vi "TCam_Calibration.vi"() -> (2 "State out":string="Data: Load Thermal Calibration")   [LabVIEW 2020]
uses:
  DataCluster_TCAL.ctl
  <vilib>/vision/Image Controls.llb/IMAQ Image.ctl
  DataCluster.ctl
  <vilib>/userDefined/High Color/IMAQdx.ctl
  <vilib>/Utility/xml.llb/Write to XML File(string).vi
panel:
  out "Pict Ring":i32(ring)
  in  "Done":bool
  out "Step":string="Step: 4\n\nCalculate temperature!"
  in  "Fixpoint Radius":i32=20 min=3 max=20
  in  "Cluster":T1 {"Points"."Top Left"."Y" format="%.2f"; "Points"."Top Left"."X" format="%.2f"; "Points"."Top Right"."Y" format="%.2f"; "Points"."Top Right"."X" format="%.2f"; "Points"."Bottom Left"."Y" format="%.2f"; "Points"."Bottom Left"."X" format="%.2f"; "Points"."Bottom Right"."Y" format="%.2f"; "Points"."Bottom Right"."X" format="%.2f"; "Points"."Fixpoint"."Y" format="%.2f"; "Points"."Fixpoint"."X" format="%.2f"}
  in  "Display Mapping":u32(ring)=10 items=["Default"=10, "Most Significant Bits"=11, "Full Dynamic"=12, "Downshift"=13, "Given Range"=14, "90% Dynamic"=15, "Given Percent Range"=16]
  in  "Image":u32(slide) scale=0.0..242.0
  in  "Help":bool
  out "Tutorial":string="Step: 4\n\nCalculate temperature!"
  in  "Show All Points":bool
  in  "Well Radius":u32=50 min=1 max=100
  in  "PCR Size":u16(ring) items=["384 (24x16)", "96 (12x8)"]
  out "Points":T3[](array[typedef])=[{"X"=103.0, "Y"=94.0}, {"X"=158.04349, "Y"=93.521736}, {"X"=213.08696, "Y"=93.04348}, {"X"=268.13043, "Y"=92.565216}, {"X"=323.17392, "Y"=92.08696}, {"X"=378.2174, "Y"=91.608696}, {"X"=433.26086, "Y"=91.13043}, {"X"=488.30435, "Y"=90.652176}, {"X"=543.34784, "Y"=90.17391}, {"X"=598.39136, "Y"=89.69565}, {"X"=653.4348, "Y"=89.21739}, {"X"=708.4783, "Y"=88.73913}, {"X"=763.5217, "Y"=88.26087}, {"X"=818.56525, "Y"=87.78261}, {"X"=873.6087, "Y"=87.30435}, {"X"=928.6522, "Y"=86.82609}, {"X"=983.6957, "Y"=86.347824}, {"X"=1038.7391, "Y"=85.86957}, {"X"=1093.7827, "Y"=85.391304}, {"X"=1148.8262, "Y"=84.91304}, {"X"=1203.8696, "Y"=84.434784}, {"X"=1258.9131, "Y"=83.95652}, {"X"=1313.9565, "Y"=83.478264}, {"X"=1369.0, "Y"=83.0}, {"X"=103.46667, "Y"=149.06667}, {"X"=158.51015, "Y"=148.58841}, {"X"=213.55362, "Y"=148.11014}, {"X"=268.5971, "Y"=147.63188}, {"X"=323.6406, "Y"=147.15363}, {"X"=378.68408, "Y"=146.67535}, {"X"=433.72754, "Y"=146.1971}, {"X"=488.77103, "Y"=145.71884}, {"X"=543.8145, "Y"=145.24057}, {"X"=598.858, "Y"=144.76231}, {"X"=653.9015, "Y"=144.28406}, {"X"=708.94495, "Y"=143.8058}, {"X"=763.9884, "Y"=143.32753}, {"X"=819.0319, "Y"=142.84927}, {"X"=874.0754, "Y"=142.37102}, {"X"=929.1189, "Y"=141.89276}, {"X"=984.16235, "Y"=141.41449}, {"X"=1039.2058, "Y"=140.93623}, {"X"=1094.2493, "Y"=140.45798}, {"X"=1149.2928, "Y"=139.9797}, {"X"=1204.3363, "Y"=139.50145}, {"X"=1259.3798, "Y"=139.0232}, {"X"=1314.4232, "Y"=138.54492}, {"X"=1369.4667, "Y"=138.06667}, {"X"=103.933334, "Y"=204.13333}, {"X"=158.9768, "Y"=203.65506}, {"X"=214.0203, "Y"=203.17682}, {"X"=269.06375, "Y"=202.69855}, {"X"=324.10724, "Y"=202.22029}, {"X"=379.15073, "Y"=201.74203}, {"X"=434.19418, "Y"=201.26376}, {"X"=489.23767, "Y"=200.7855}, {"X"=544.2812, "Y"=200.30725}, {"X"=599.32465, "Y"=199.82898}, {"X"=654.36816, "Y"=199.35072}, {"X"=709.4116, "Y"=198.87247}, {"X"=764.4551, "Y"=198.3942}, {"X"=819.4986, "Y"=197.91594}, {"X"=874.54205, "Y"=197.43768}, {"X"=929.5856, "Y"=196.95941}, {"X"=984.629, "Y"=196.48116}, {"X"=1039.6725, "Y"=196.0029}, {"X"=1094.716, "Y"=195.52463}, {"X"=1149.7595, "Y"=195.04637}, {"X"=1204.803, "Y"=194.56812}, {"X"=1259.8464, "Y"=194.08984}, {"X"=1314.8899, "Y"=193.6116}, {"X"=1369.9333, "Y"=193.13333}, {"X"=104.4, "Y"=259.2}, {"X"=159.44348, "Y"=258.72174}, {"X"=214.48695, "Y"=258.24347}, {"X"=269.53043, "Y"=257.7652}, {"X"=324.5739, "Y"=257.28696}, {"X"=379.6174, "Y"=256.8087}, {"X"=434.66086, "Y"=256.33044}, {"X"=489.70435, "Y"=255.85217}, {"X"=544.74786, "Y"=255.37392}, {"X"=599.7913, "Y"=254.89565}, {"X"=654.83484, "Y"=254.41739}, {"X"=709.8783, "Y"=253.93913}, {"X"=764.92175, "Y"=253.46086}, {"X"=819.9653, "Y"=252.9826}, {"X"=875.0087, "Y"=252.50435}, {"X"=930.05225, "Y"=252.02608}, {"X"=985.0957, "Y"=251.54782}, {"X"=1040.1392, "Y"=251.06956}, {"X"=1095.1826, "Y"=250.59131}, {"X"=1150.2262, "Y"=250.11304}, {"X"=1205.2697, "Y"=249.63478}, {"X"=1260.3131, "Y"=249.15652}, {"X"=1315.3566, "Y"=248.67825}, {"X"=1370.4, "Y"=248.2}, {"X"=104.86667, "Y"=314.26666}, {"X"=159.91014, "Y"=313.7884}, {"X"=214.95363, "Y"=313.31012}, {"X"=269.9971, "Y"=312.83188}, {"X"=325.0406, "Y"=312.35364}, {"X"=380.08408, "Y"=311.87537}, {"X"=435.12753, "Y"=311.3971}, {"X"=490.17102, "Y"=310.91882}, {"X"=545.2145, "Y"=310.44058}, {"X"=600.258, "Y"=309.9623}, {"X"=655.30145, "Y"=309.48407}, {"X"=710.3449, "Y"=309.0058}, {"X"=765.38837, "Y"=308.52753}, {"X"=820.4319, "Y"=308.04926}, {"X"=875.47534, "Y"=307.571}, {"X"=930.51886, "Y"=307.09274}, {"X"=985.5623, "Y"=306.6145}, {"X"=1040.6058, "Y"=306.13623}, {"X"=1095.6493, "Y"=305.65796}, {"X"=1150.6929, "Y"=305.1797}, {"X"=1205.7363, "Y"=304.70145}, {"X"=1260.7798, "Y"=304.2232}, {"X"=1315.8232, "Y"=303.74493}, {"X"=1370.8667, "Y"=303.26666}, {"X"=105.333336, "Y"=369.3333}, {"X"=160.37682, "Y"=368.85504}, {"X"=215.42029, "Y"=368.3768}, {"X"=270.46378, "Y"=367.89853}, {"X"=325.50726, "Y"=367.42026}, {"X"=380.55075, "Y"=366.94202}, {"X"=435.5942, "Y"=366.46375}, {"X"=490.6377, "Y"=365.98547}, {"X"=545.68115, "Y"=365.50723}, {"X"=600.7247, "Y"=365.02896}, {"X"=655.7681, "Y"=364.5507}, {"X"=710.8116, "Y"=364.07245}, {"X"=765.85504, "Y"=363.59418}, {"X"=820.89856, "Y"=363.11594}, {"X"=875.942, "Y"=362.63766}, {"X"=930.98553, "Y"=362.1594}, {"X"=986.029, "Y"=361.68115}, {"X"=1041.0725, "Y"=361.20288}, {"X"=1096.116, "Y"=360.7246}, {"X"=1151.1595, "Y"=360.24637}, {"X"=1206.203, "Y"=359.7681}, {"X"=1261.2465, "Y"=359.28983}, {"X"=1316.2899, "Y"=358.81158}, {"X"=1371.3334, "Y"=358.3333}, {"X"=105.8, "Y"=424.4}, {"X"=160.84348, "Y"=423.92172}, {"X"=215.88696, "Y"=423.44348}, {"X"=270.93042, "Y"=422.9652}, {"X"=325.9739, "Y"=422.48694}, {"X"=381.0174, "Y"=422.0087}, {"X"=436.06085, "Y"=421.53043}, {"X"=491.10434, "Y"=421.05215}, {"X"=546.1478, "Y"=420.5739}, {"X"=601.19135, "Y"=420.09564}, {"X"=656.2348, "Y"=419.61737}, {"X"=711.27826, "Y"=419.13913}, {"X"=766.3217, "Y"=418.66086}, {"X"=821.36523, "Y"=418.18262}, {"X"=876.4087, "Y"=417.70435}, {"X"=931.4522, "Y"=417.22607}, {"X"=986.49567, "Y"=416.74783}, {"X"=1041.5392, "Y"=416.26956}, {"X"=1096.5826, "Y"=415.7913}, {"X"=1151.6262, "Y"=415.31305}, {"X"=1206.6697, "Y"=414.83478}, {"X"=1261.7131, "Y"=414.3565}, {"X"=1316.7566, "Y"=413.87827}, {"X"=1371.8, "Y"=413.4}, {"X"=106.26667, "Y"=479.46667}, {"X"=161.31015, "Y"=478.9884}, {"X"=216.35362, "Y"=478.51016}, {"X"=271.3971, "Y"=478.0319}, {"X"=326.44058, "Y"=477.55362}, {"X"=381.48407, "Y"=477.07538}, {"X"=436.52753, "Y"=476.5971}, {"X"=491.571, "Y"=476.11884}, {"X"=546.6145, "Y"=475.6406}, {"X"=601.658, "Y"=475.16232}, {"X"=656.7015, "Y"=474.68405}, {"X"=711.74493, "Y"=474.2058}, {"X"=766.7884, "Y"=473.72754}, {"X"=821.8319, "Y"=473.2493}, {"X"=876.87537, "Y"=472.77103}, {"X"=931.9189, "Y"=472.29276}, {"X"=986.96234, "Y"=471.8145}, {"X"=1042.0059, "Y"=471.33624}, {"X"=1097.0493, "Y"=470.85797}, {"X"=1152.0929, "Y"=470.37973}, {"X"=1207.1364, "Y"=469.90146}, {"X"=1262.1798, "Y"=469.4232}, {"X"=1317.2233, "Y"=468.94495}, {"X"=1372.2667, "Y"=468.46667}, {"X"=106.73333, "Y"=534.5333}, {"X"=161.77681, "Y"=534.05505}, {"X"=216.8203, "Y"=533.5768}, {"X"=271.86377, "Y"=533.0985}, {"X"=326.90726, "Y"=532.62024}, {"X"=381.95074, "Y"=532.142}, {"X"=436.9942, "Y"=531.66376}, {"X"=492.0377, "Y"=531.1855}, {"X"=547.0812, "Y"=530.7073}, {"X"=602.12463, "Y"=530.229}, {"X"=657.16815, "Y"=529.75073}, {"X"=712.2116, "Y"=529.27246}, {"X"=767.25507, "Y"=528.7942}, {"X"=822.2986, "Y"=528.3159}, {"X"=877.34204, "Y"=527.83765}, {"X"=932.38556, "Y"=527.3594}, {"X"=987.429, "Y"=526.88116}, {"X"=1042.4724, "Y"=526.4029}, {"X"=1097.516, "Y"=525.9246}, {"X"=1152.5594, "Y"=525.4464}, {"X"=1207.6029, "Y"=524.96814}, {"X"=1262.6464, "Y"=524.48987}, {"X"=1317.6898, "Y"=524.0116}, {"X"=1372.7333, "Y"=523.5333}, {"X"=107.2, "Y"=589.6}, {"X"=162.24348, "Y"=589.1217}, {"X"=217.28696, "Y"=588.64343}, {"X"=272.33044, "Y"=588.16516}, {"X"=327.37393, "Y"=587.6869}, {"X"=382.41742, "Y"=587.2087}, {"X"=437.46088, "Y"=586.7304}, {"X"=492.50436, "Y"=586.25214}, {"X"=547.54785, "Y"=585.7739}, {"X"=602.5913, "Y"=585.29565}, {"X"=657.6348, "Y"=584.8174}, {"X"=712.6783, "Y"=584.3391}, {"X"=767.72174, "Y"=583.86084}, {"X"=822.76526, "Y"=583.38257}, {"X"=877.8087, "Y"=582.9043}, {"X"=932.85223, "Y"=582.426}, {"X"=987.8957, "Y"=581.9478}, {"X"=1042.9391, "Y"=581.46954}, {"X"=1097.9827, "Y"=580.9913}, {"X"=1153.0261, "Y"=580.51306}, {"X"=1208.0696, "Y"=580.0348}, {"X"=1263.113, "Y"=579.5565}, {"X"=1318.1565, "Y"=579.07825}, {"X"=1373.2, "Y"=578.6}, {"X"=107.666664, "Y"=644.6666}, {"X"=162.71014, "Y"=644.18835}, {"X"=217.75363, "Y"=643.7101}, {"X"=272.7971, "Y"=643.2319}, {"X"=327.84058, "Y"=642.7536}, {"X"=382.88406, "Y"=642.2753}, {"X"=437.92752, "Y"=641.79706}, {"X"=492.971, "Y"=641.3188}, {"X"=548.0145, "Y"=640.8405}, {"X"=603.058, "Y"=640.3623}, {"X"=658.1015, "Y"=639.88403}, {"X"=713.14496, "Y"=639.40576}, {"X"=768.1884, "Y"=638.9275}, {"X"=823.23193, "Y"=638.4492}, {"X"=878.2754, "Y"=637.97095}, {"X"=933.3189, "Y"=637.49274}, {"X"=988.36237, "Y"=637.01447}, {"X"=1043.4058, "Y"=636.5362}, {"X"=1098.4493, "Y"=636.0579}, {"X"=1153.4928, "Y"=635.57965}, {"X"=1208.5363, "Y"=635.1014}, {"X"=1263.5797, "Y"=634.62317}, {"X"=1318.6232, "Y"=634.1449}, {"X"=1373.6666, "Y"=633.6666}, {"X"=108.13333, "Y"=699.73334}, {"X"=163.17682, "Y"=699.25507}, {"X"=218.22029, "Y"=698.7768}, {"X"=273.26376, "Y"=698.2986}, {"X"=328.30725, "Y"=697.8203}, {"X"=383.35074, "Y"=697.34204}, {"X"=438.3942, "Y"=696.8638}, {"X"=493.43768, "Y"=696.3855}, {"X"=548.4812, "Y"=695.9072}, {"X"=603.52466, "Y"=695.429}, {"X"=658.5682, "Y"=694.95074}, {"X"=713.61163, "Y"=694.4725}, {"X"=768.6551, "Y"=693.9942}, {"X"=823.6986, "Y"=693.5159}, {"X"=878.74207, "Y"=693.03766}, {"X"=933.7856, "Y"=692.55945}, {"X"=988.82904, "Y"=692.0812}, {"X"=1043.8724, "Y"=691.6029}, {"X"=1098.916, "Y"=691.12463}, {"X"=1153.9595, "Y"=690.64636}, {"X"=1209.0029, "Y"=690.1681}, {"X"=1264.0464, "Y"=689.6899}, {"X"=1319.0898, "Y"=689.2116}, {"X"=1374.1333, "Y"=688.73334}, {"X"=108.6, "Y"=754.8}, {"X"=163.64348, "Y"=754.3217}, {"X"=218.68697, "Y"=753.84344}, {"X"=273.73044, "Y"=753.36523}, {"X"=328.77393, "Y"=752.88696}, {"X"=383.8174, "Y"=752.4087}, {"X"=438.86087, "Y"=751.9304}, {"X"=493.90436, "Y"=751.45215}, {"X"=548.9478, "Y"=750.9739}, {"X"=603.99133, "Y"=750.49567}, {"X"=659.0348, "Y"=750.0174}, {"X"=714.07825, "Y"=749.5391}, {"X"=769.1217, "Y"=749.06085}, {"X"=824.1652, "Y"=748.5826}, {"X"=879.2087, "Y"=748.1043}, {"X"=934.2522, "Y"=747.6261}, {"X"=989.29565, "Y"=747.1478}, {"X"=1044.3391, "Y"=746.66956}, {"X"=1099.3827, "Y"=746.1913}, {"X"=1154.4261, "Y"=745.713}, {"X"=1209.4696, "Y"=745.23474}, {"X"=1264.5131, "Y"=744.75653}, {"X"=1319.5565, "Y"=744.27826}, {"X"=1374.6, "Y"=743.8}, {"X"=109.066666, "Y"=809.86664}, {"X"=164.11015, "Y"=809.38837}, {"X"=219.15363, "Y"=808.9101}, {"X"=274.1971, "Y"=808.4319}, {"X"=329.2406, "Y"=807.9536}, {"X"=384.2841, "Y"=807.47534}, {"X"=439.32755, "Y"=806.9971}, {"X"=494.37103, "Y"=806.5188}, {"X"=549.4145, "Y"=806.0405}, {"X"=604.458, "Y"=805.5623}, {"X"=659.50146, "Y"=805.08405}, {"X"=714.5449, "Y"=804.6058}, {"X"=769.5884, "Y"=804.1275}, {"X"=824.6319, "Y"=803.64923}, {"X"=879.67535, "Y"=803.17096}, {"X"=934.7189, "Y"=802.69275}, {"X"=989.7623, "Y"=802.2145}, {"X"=1044.8058, "Y"=801.7362}, {"X"=1099.8494, "Y"=801.25793}, {"X"=1154.8928, "Y"=800.77966}, {"X"=1209.9363, "Y"=800.3014}, {"X"=1264.9797, "Y"=799.8232}, {"X"=1320.0232, "Y"=799.3449}, {"X"=1375.0667, "Y"=798.86664}, {"X"=109.53333, "Y"=864.93335}, {"X"=164.57681, "Y"=864.4551}, {"X"=219.6203, "Y"=863.9768}, {"X"=274.66376, "Y"=863.4986}, {"X"=329.70724, "Y"=863.0203}, {"X"=384.75073, "Y"=862.54205}, {"X"=439.7942, "Y"=862.0638}, {"X"=494.83768, "Y"=861.5855}, {"X"=549.88116, "Y"=861.10724}, {"X"=604.9247, "Y"=860.629}, {"X"=659.96814, "Y"=860.15076}, {"X"=715.0116, "Y"=859.6725}, {"X"=770.05505, "Y"=859.1942}, {"X"=825.0986, "Y"=858.71594}, {"X"=880.142, "Y"=858.2377}, {"X"=935.18555, "Y"=857.75946}, {"X"=990.229, "Y"=857.2812}, {"X"=1045.2725, "Y"=856.8029}, {"X"=1100.316, "Y"=856.32465}, {"X"=1155.3595, "Y"=855.8464}, {"X"=1210.403, "Y"=855.3681}, {"X"=1265.4464, "Y"=854.8899}, {"X"=1320.4899, "Y"=854.4116}, {"X"=1375.5333, "Y"=853.93335}, {"X"=110.0, "Y"=920.0}, {"X"=165.04349, "Y"=919.5217}, {"X"=220.08696, "Y"=919.04346}, {"X"=275.13043, "Y"=918.56525}, {"X"=330.17392, "Y"=918.087}, {"X"=385.2174, "Y"=917.6087}, {"X"=440.26086, "Y"=917.13043}, {"X"=495.30435, "Y"=916.65216}, {"X"=550.34784, "Y"=916.1739}, {"X"=605.39136, "Y"=915.6957}, {"X"=660.4348, "Y"=915.2174}, {"X"=715.4783, "Y"=914.73914}, {"X"=770.5217, "Y"=914.26086}, {"X"=825.56525, "Y"=913.7826}, {"X"=880.6087, "Y"=913.3043}, {"X"=935.6522, "Y"=912.8261}, {"X"=990.6957, "Y"=912.34784}, {"X"=1045.7391, "Y"=911.86957}, {"X"=1100.7827, "Y"=911.3913}, {"X"=1155.8262, "Y"=910.913}, {"X"=1210.8696, "Y"=910.43475}, {"X"=1265.9131, "Y"=909.95654}, {"X"=1320.9565, "Y"=909.4783}, {"X"=1376.0, "Y"=909.0}] {"Y" format="%.2f"; "X" format="%.2f"}
  out "State":i32=3
  in  "Previous":bool
  in  "Next":bool
  in  "Path":path caption="Image Path"
  out "Image":T2(plugin-control)
  # "hints \nPress F1 or F2 to cycle through the steps\nUse the Mouse Wheel to zoom in and out"
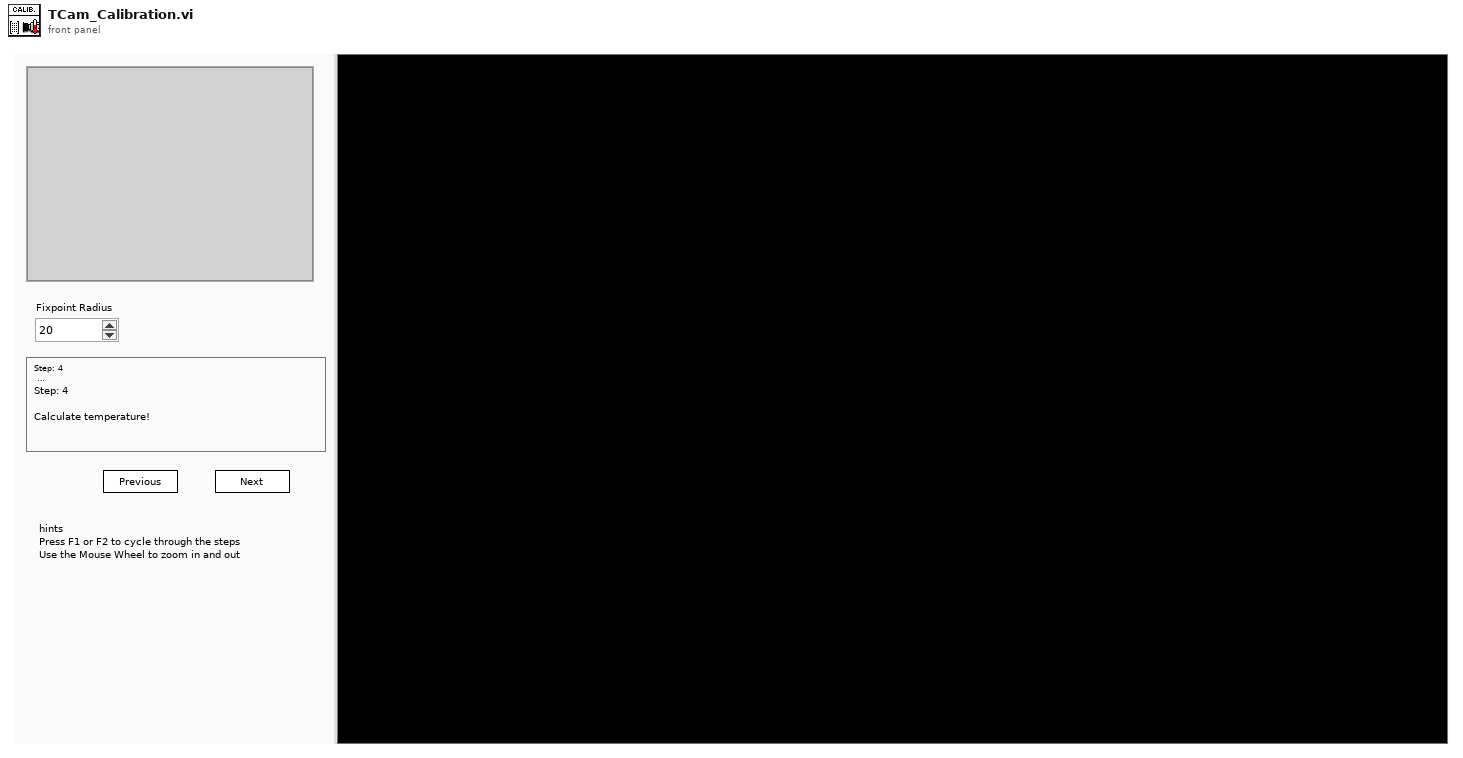
[diagram p1: front panel]
types:
  T1 = typedef "DataCluster_TCAL.ctl" = cluster{"Core":cluster{"Current VI Reference":refnum<vi>, "Close Panel on Exit?":bool}, "Image Out":T2, "State":i32, "Points":cluster{"Top Left":T3, "Top Right":T3, "Bottom Left":T3, "Bottom Right":T3, "x space 2":dbl, "y space 2":sgl, "x_space":sgl, "y_space":sgl, "Pixels":cluster{"X":i32, "Y":i32}[][], "Fixpoint":T3}, "img_array":T2[], "Temps":dbl[], "Temps_Array":dbl[][]}
  T2 = typedef "IMAQ Image.ctl" = refnum<image>
  T3 = typedef "IMAQ Point" = cluster{"X":sgl, "Y":sgl}
  T4 = enum32{"Invalid", "Standard", "Closed", "Hidden", "Minimized", "Maximized"}
  T5 = enum32{"invalid app kind", "Development System", "Run Time System", "Student Edition", "Embedded LabVIEW", "Evaluation", "Custom"}
  T6 = cluster{"Global Rectangle":i32[], "Contours":cluster{"Contour Type":u32, "ROI Type":u32, "Points":i32[]}[]}
  T7 = typedef "DataCluster.ctl" = cluster{"Core":cluster{"Current VI Reference":refnum<vi>, "Close Panel on Exit?":bool, "Exit":bool, "Initialized?":bool}, "Connections":cluster{"cDAQ Therm":cluster{"Task":refnum<k21>, "Connected":bool, "Active":bool}, "cDAQ Voltage":cluster{"Task":refnum<k21>, "Connected":bool, "Active":bool}, "cDAQ ID":string, "Camera":cluster{"Session":T8, "Connected":bool, "Active":bool, "Placeholder":T2}, "PSU":cluster{"Port":refnum<visa-resource-name>, "Connected":bool, "Active":bool}}, "Data Acquisition":cluster{"Setup":cluster{"Label":string, "Operator":string, "Notes":string, "TempGrad":dbl, "TargetTemp":dbl, "Sample Volume":dbl}, "Camera":cluster{"Image":T2, "Save Image":T2, "Image Frequency":i32, "Rectangle":T9, "Calibration":cluster{"Top Left":T3, "Top Right":T3, "Bottom Left":T3, "Bottom Right":T3, "Fixpoint":T3, "Scan Area":dbl, "Fixpoint Area":dbl, "Well Pixels":cluster{"X":i32, "Y":i32}[][], "Valid":bool}, "FocusPos":u32, "Display Mapping":u32}, "Thermistor":cluster{"Sample Size":i32, "Calibration":cluster{"B0.100":dbl[], "R25":dbl[], "c":dbl[][], "State":bool[], "V_S":dbl, "R_S":dbl}, "Timing Mode":i32}, "Partition":cluster{"Data":string[][], "Cell Label":string, "Cell Color":u32, "Height":i32, "Width":i32, "Grid":string[][]}, "Queue":cluster{"Size":i32, "Queue":refnum<queue>}, "Sample Rate":i32, "Active":bool, "Ready":bool, "Graph Mode":u16}, "Control":cluster{"Sample Rate":i32, "PID gains":cluster{"proportional gain (Kc)":dbl, "integral time (Ti, min)":dbl, "derivative time (Td, min)":dbl}}}
  T8 = typedef "IMAQdx.ctl" = refnum<k21>
  T9 = typedef "IMAQ Rectangle" = cluster{"Left":i32, "Top":i32, "Right":i32, "Bottom":i32, "Rotation":dbl}
  T10 = enum16{"open", "replace", "create", "open or create", "replace or create", "replace or create with confirmation"}
  T11 = typedef "ROI Descriptor" = cluster{"Global Rectangle":i32[], "Contours":cluster{"ID":enum32{"External", "Internal"}, "Type":u32, "Coordinates":i32[]}[]}
  T12 = typedef "Image Type" = u32
  T13 = cluster{"Current VI Reference":refnum<vi>, "Close Panel on Exit?":bool}
  T14 = cluster{"Top Left":T3, "Top Right":T3, "Bottom Left":T3, "Bottom Right":T3, "x space 2":dbl, "y space 2":sgl, "x_space":sgl, "y_space":sgl, "Pixels":cluster{"X":i32, "Y":i32}[][], "Fixpoint":T3}
  T15 = cluster{"Core":cluster{"Current VI Reference":refnum<vi>, "Close Panel on Exit?":bool}, "Image Out":T2, "State":i32, "Points":cluster{"Top Left":T3, "Top Right":T3, "Bottom Left":T3, "Bottom Right":T3, "x space 2":dbl, "y space 2":sgl, "x_space":sgl, "y_space":sgl, "Pixels":cluster{"X":i32, "Y":i32}[][], "Fixpoint":T3}, "img_array":T2[], "Temps":dbl[], "Temps_Array":dbl[][]}
  T16 = cluster{"Top Left":T3, "Top Right":T3, "Bottom Left":T3, "Bottom Right":T3, "Fixpoint":T3, "Scan Area":dbl, "Fixpoint Area":dbl, "Well Pixels":cluster{"X":i32, "Y":i32}[][], "Valid":bool}
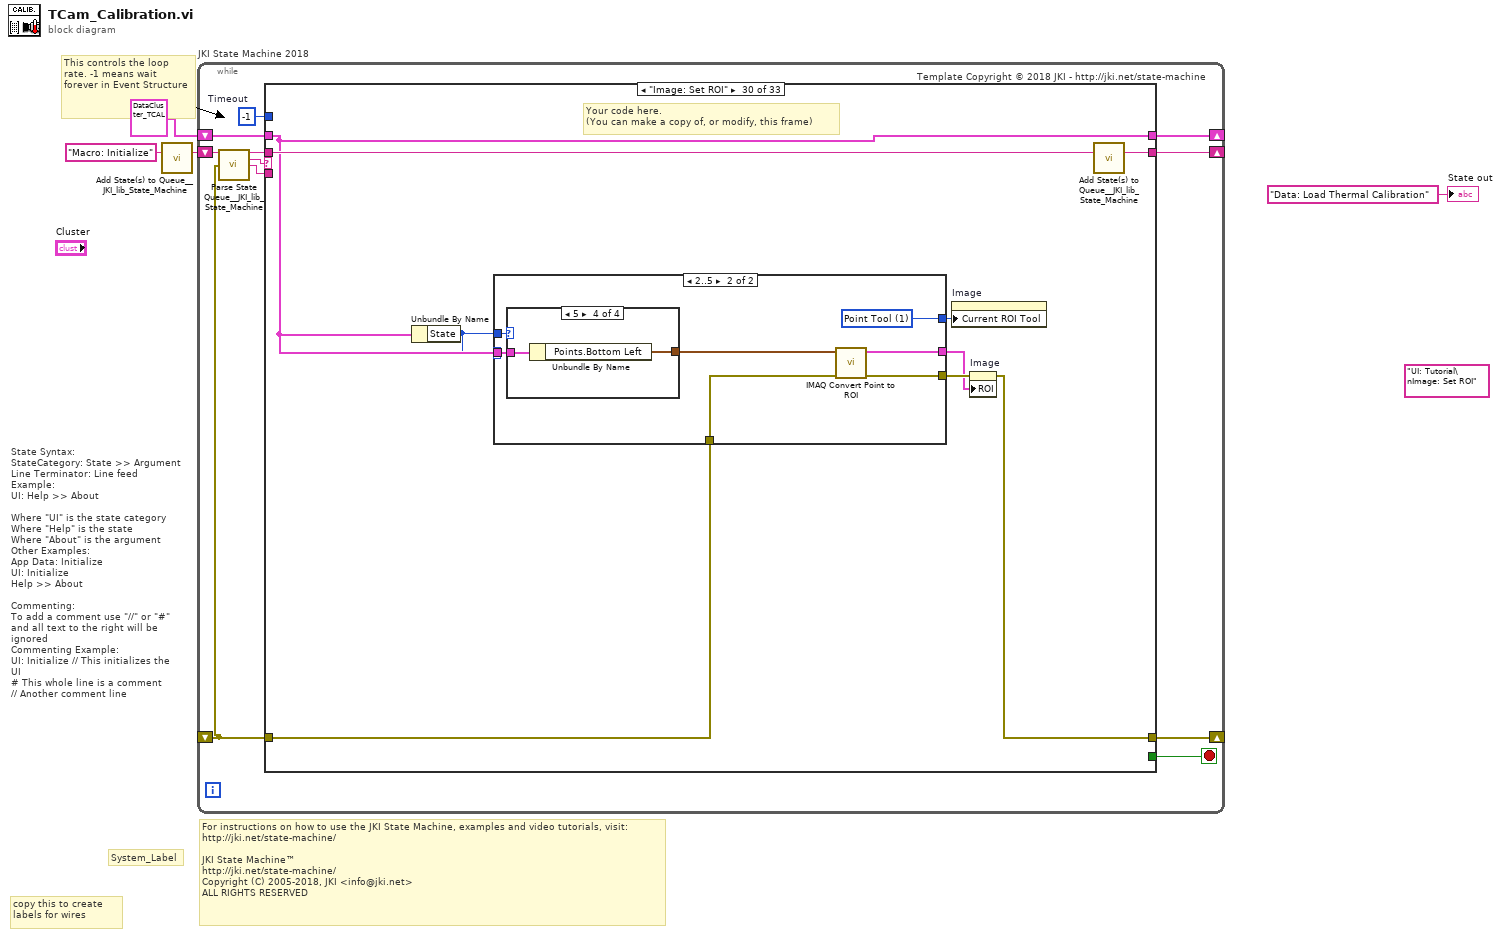
[diagram p0: block diagram]
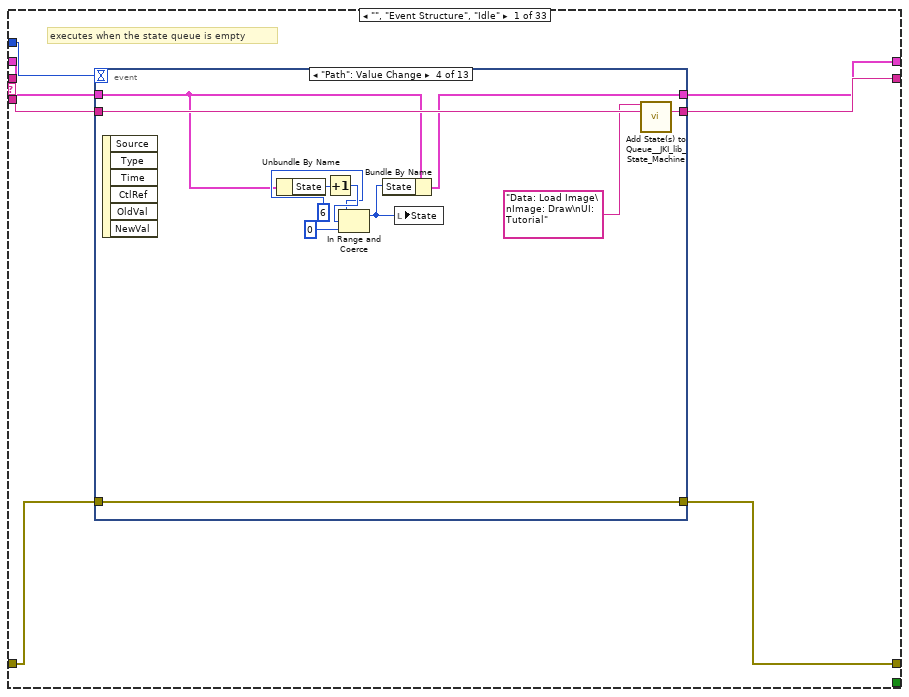
[diagram p2: hidden frame]
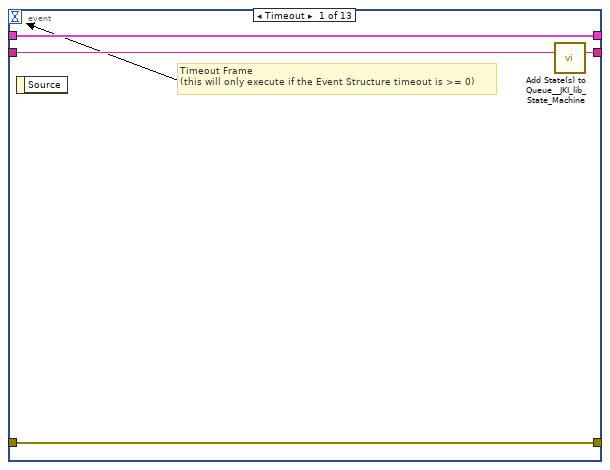
[diagram p3: hidden frame]
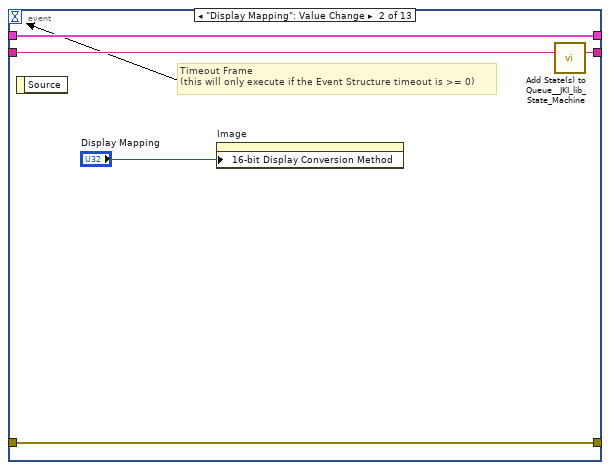
[diagram p4: hidden frame]
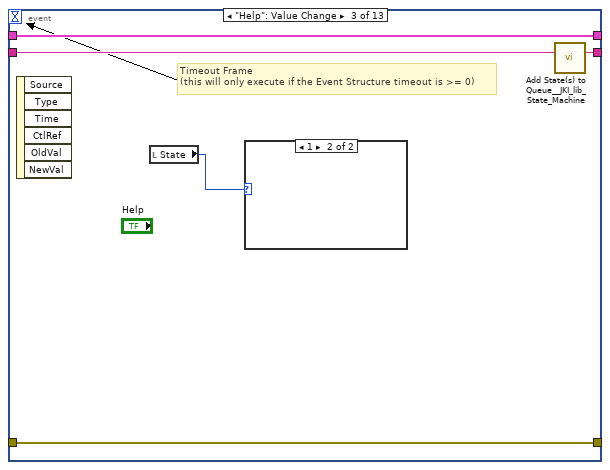
[diagram p5: hidden frame]
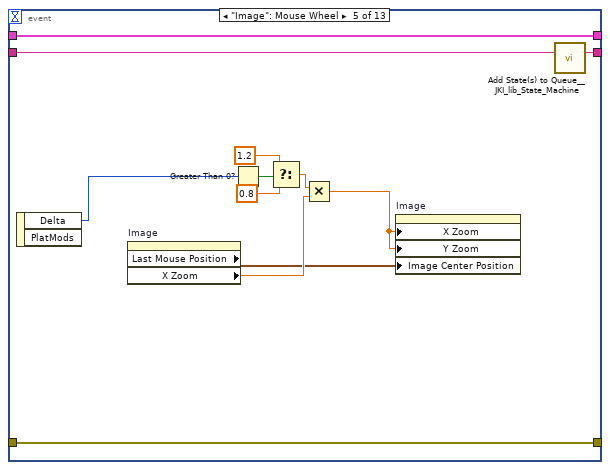
[diagram p7: hidden frame]
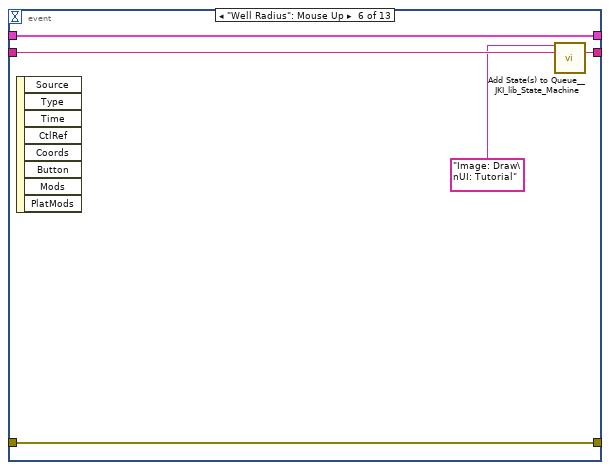
[diagram p8: hidden frame]
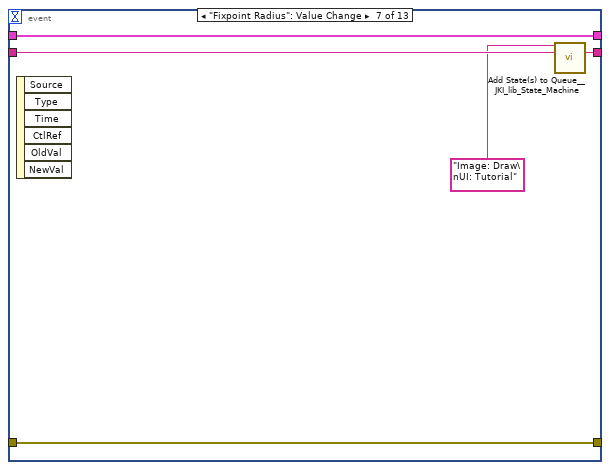
[diagram p9: hidden frame]
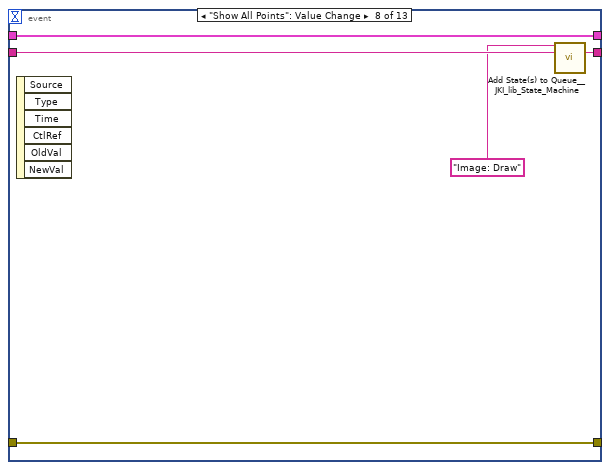
[diagram p10: hidden frame]
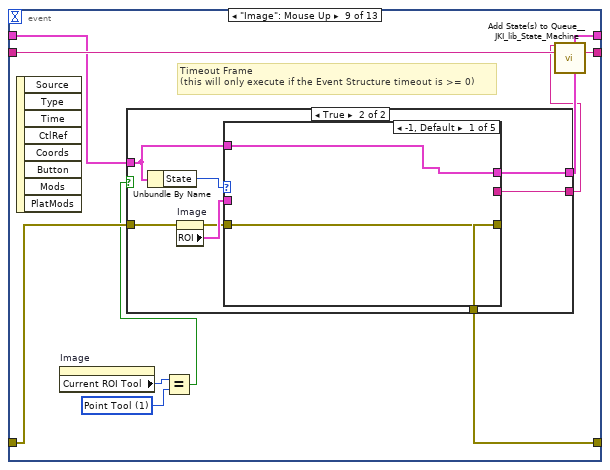
[diagram p11: hidden frame]
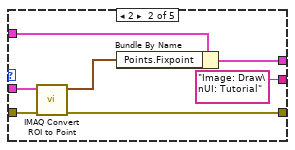
[diagram p13: hidden frame]
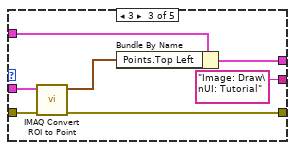
[diagram p14: hidden frame]
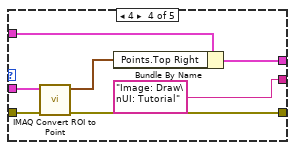
[diagram p15: hidden frame]
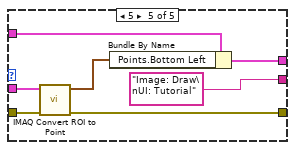
[diagram p16: hidden frame]
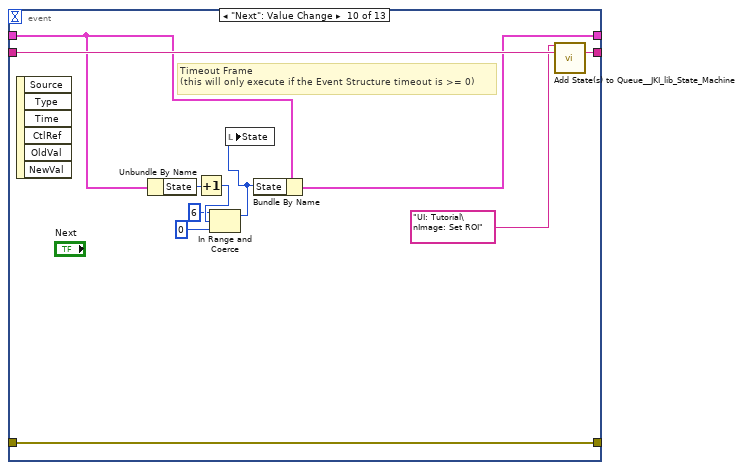
[diagram p17: hidden frame]
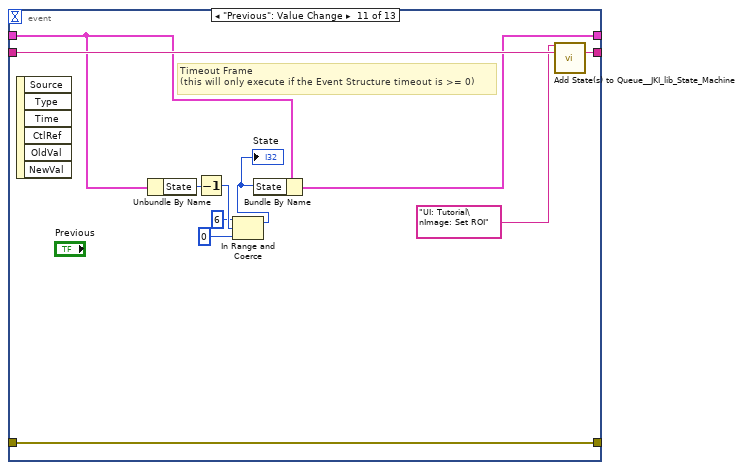
[diagram p18: hidden frame]
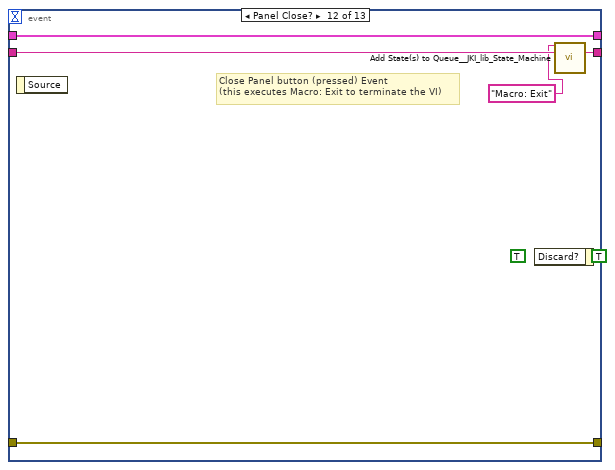
[diagram p19: hidden frame]
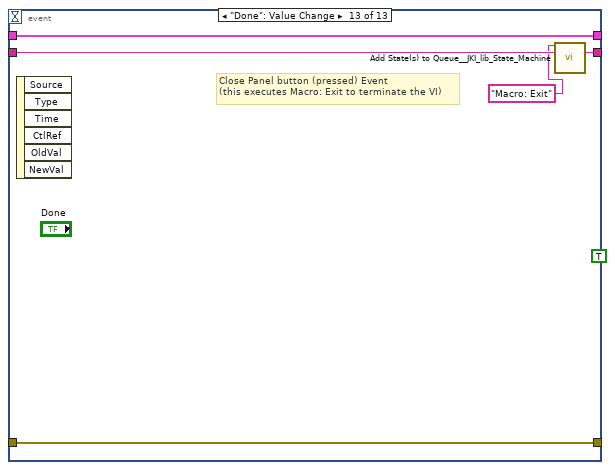
[diagram p20: hidden frame]
diagram:
  (unwired) "UI: Tutorial\nImage: Set ROI" ("f")
  # "For instructions on how to use the JKI State Machine, examples and video tutorials, visit:\nhttp://jki.net/state-machine/\n\nJKI State Machine™\nhttp://jki.net/state-machine/\nCopyright (C) 2005-2018, JKI <info@jki.net>\nALL RIGHTS RESERVED"
  # "State Syntax:\nStateCategory: State >> Argument\nLine Terminator: Line feed\nExample:\nUI: Help >> About\n\nWhere \"UI\" is the state category\nWhere \"Help\" is the state\nWhere \"About\" is the argument\nOther Examples:\nApp Data: Initialize\nUI: Initialize\nHelp >> About\n\nCommenting:\nTo add a comment use \"//\" or \"#\" and all text to the right will be ignored\nCommenting Example:\nUI: Initialize // This initializes the UI\n# This whole line is a comment\n// Another comment line"
  # "copy this to create labels for wires"
  # "This controls the loop rate. -1 means wait forever in Event Structure"
  # "System_Label"
  n1 = call <vilib>:"Add State(s) to Queue__JKI_lib_State_Machine.vi"("State(s) in (\"\")"="Macro: Initialize") -> ("States Out"=w4:string)  [unwired: 14 in]
  n2 = while "JKI State Machine 2018" {
    shift-right: [w8] -> _
    shift-left: T1 {"Core"={"Current VI Reference"=refnum, "Close Panel on Exit?"=FALSE}, "Image Out"=refnum, "State"=0, "Points"={"Top Left"={"X"=0.0, "Y"=0.0}, "Top Right"={"X"=0.0, "Y"=0.0}, "Bottom Left"={"X"=0.0, "Y"=0.0}, "Bottom Right"={"X"=0.0, "Y"=0.0}, "x space 2"=0.0, "y space 2"=0.0, "x_space"=0.0, "y_space"=0.0, "Pixels"=[], "Fixpoint"={"X"=0.0, "Y"=0.0}}, "img_array"=[], "Temps"=[], "Temps_Array"=[]} ("output cluster") -> [w7]
    shift-right: [w11] -> _
    shift-left: _ -> [w5]
    shift-right: [w10] -> _
    shift-left: w4 -> [w12]
    stop <- w9 stop-if-true
    w6 = -1  # Timeout
    # "Template Copyright © 2018 JKI - http://jki.net/state-machine"
    n3 = call <vilib>:"Parse State Queue__JKI_lib_State_Machine.vi"("State Queue"=w12, "Error In (no error)"=w5) -> ("Remaining States"=w14:string, "Current State"=w15:string, "Arguments"=w13:string)  [unwired: 11 in]
    n4 = case shown="\"Image: Set ROI\"" w15 {
      selector: w15 -> [_ _ w162 _ _ _ _ _ _ _ _ _ _ _ _ _ _ _ _ _ _ _ _ _ _ _ _ _ _ _ _ _ _]
      tunnel: w14 -> [w22 w161 w166 w185 w191 w196 w200 w209 w230 w235 w249 w282 w292 w312 w330 w386 w397 w466 w471 w481 w485 w490 w495 w515 w532 w538 w556 w576 w594 w605 w633 w700 w722]
      tunnel: w13 -> [_ _ _ _ _ _ _ _ _ _ _ _ _ _ _ w381 w391 _ _ _ _ _ _ _ _ _ _ _ _ _ w631 _ _]
      tunnel: w7 -> [w20 w158 w164 w178 w188 w194 w197 w207 w227 w231 _ w279 w289 w310 w317 w384 w393 w463 w468 w478 w482 w487 w492 w496 w530 w536 w547 w567 w585 w603 w629 w687 w711]
      tunnel: [w19 w159 w168 w182 errorcluster {"status"=FALSE, "code"=0, "source"=""} ("error out") w193 w198 w201 w224 w233 w240 w276 w290 w309 w328 w382 w394 w464 w469 w479 w483 w488 w493 w513 w525 w533 w554 w574 w592 w598 w626 w697 w720] -> w11
      tunnel: w5 -> [w18 w159 w167 w182 w187 w193 w198 w205 w224 w233 w241 w264 w290 w309 w328 w383 w395 w464 w469 w479 w483 w488 w493 w513 w525 w534 w554 w574 w592 w602 w627 w697 w720]
      tunnel: [w21 w160 w165 w184 w190 w195 w199 w208 w229 w234 w248 w281 w291 w311 w329 w385 w396 w465 w470 w480 w484 w489 w494 w514 w531 w537 w555 w575 w593 w604 w632 w699 w721] -> w10
      tunnel: [_ _ _ _ _ TRUE _ _ _ _ _ _ _ _ _ _ _ _ _ _ _ _ _ _ _ _ _ _ _ _ _ _ _] -> w9
      tunnel: [w17 w158 w164 w183 w188 w194 w197 w206 w228 w231 w247 w279 w289 w310 w317 w384 w393 w463 w468 w478 w482 w487 w492 w496 w530 w536 w546 w566 w584 w603 w629 w686 w711] -> w8
      tunnel: w6 -> [w16 _ _ _ _ _ _ _ _ _ _ _ _ _ _ _ _ _ _ _ _ _ _ _ _ _ _ _ _ _ _ _ _]
      frame "", "Event Structure", "Idle" {
        # "executes when the state queue is empty"
        n5 = event shown="[3] \"Path\": Value Change" {
          selector: _ -> [_ _ _ _ _ _ _ _ _ _ _ _ _]
          dyn-events: _ -> [_ _ _ _ _ _ _ _ _ _ _ _ _]
          timeout: w16 -> [_ _ _ _ _ _ _ _ _ _ _ _ _]
          tunnel: w22 -> [w26 w31 w36 w47 w59 w64 w69 w74 w84 w135 w146 w152 w157]
          tunnel: [w25 w30 w35 w46 w58 w63 w68 w73 w83 w134 w145 w151 w156] -> w21
          tunnel: w20 -> [w23 w28 w33 w38 w56 w61 w66 w71 w81 w133 w144 w149 w154]
          tunnel: [w24 w29 w34 w45 w57 w62 w67 w72 w79 w130 w141 w150 w155] -> w19
          tunnel: w18 -> [w24 w29 w34 w45 w57 w62 w67 w72 w82 w130 w141 w150 w155]
          tunnel: [w23 w28 w33 w39 w56 w61 w66 w71 w80 w131 w142 w149 w154] -> w17
          event Timeout {
            # "Timeout Frame\n(this will only execute if the Event Structure timeout is >= 0)"
            n6 = event-data() -> ()  [unwired: 1 in, 1 out]
            n7 = call <vilib>:"Add State(s) to Queue__JKI_lib_State_Machine.vi"("State(s) in (\"\")"=w26) -> ("States Out"=w25:string)  [unwired: 14 in]
          }
          event "Display Mapping": Value Change {
            # "Timeout Frame\n(this will only execute if the Event Structure timeout is >= 0)"
            n8 = event-data() -> ()  [unwired: 1 in, 1 out]
            n9 = property on="Image" class="ImageControl"("16-bit Display Conversion Method"="Display Mapping") -> ()  [unwired: 2 in, 2 out]
            n10 = call <vilib>:"Add State(s) to Queue__JKI_lib_State_Machine.vi"("State(s) in (\"\")"=w31) -> ("States Out"=w30:string)  [unwired: 14 in]
          }
          event "Help": Value Change {
            # "Timeout Frame\n(this will only execute if the Event Structure timeout is >= 0)"
            n11 = event-data() -> ()  [unwired: 1 in, 6 out]
            n12 = local read "State"() -> (w32:i32)
            n13 = case shown="1" w32 {
              frame 0, Default {
              }
              frame 1 {
              }
            }
            n14 = call <vilib>:"Add State(s) to Queue__JKI_lib_State_Machine.vi"("State(s) in (\"\")"=w36) -> ("States Out"=w35:string)  [unwired: 14 in]
          }
          event "Path": Value Change {
            n15 = event-data() -> ()  [unwired: 1 in, 6 out]
            n16 = Unbundle By Name(w38) -> ("State"=w43:i32)
            n17 = Increment(x=w43) -> (x+1=w42:i32)
            n18 = In Range and Coerce(upper limit=6, x=w42, lower limit=0) -> (coerced(x)=w37:i32)  [unwired: 1 out]
            n19 = Bundle By Name(cluster=w38, "State"=w37) -> (w39:T1)
            n20 = local write "State"(w37) -> ()
            n21 = call <vilib>:"Add State(s) to Queue__JKI_lib_State_Machine.vi"("State(s) in Front (\"\")"="Data: Load Image\nImage: Draw\nUI: Tutorial" ("State(s) in Front (\"\")"), "State(s) in (\"\")"=w47) -> ("States Out"=w46:string)  [unwired: 13 in]
          }
          event "Image": Mouse Wheel {
            n22 = event-data() -> ("Delta"=w55:i32)  [unwired: 1 in, 1 out]
            n23 = property on="Image" class="ImageControl"() -> ("Last Mouse Position"=w49:cluster{"X":i32, "Y":i32}, "X Zoom"=w50:sgl)  [unwired: 2 in, 2 out]
            n24 = Greater Than 0?(x=w55) -> (x > 0?=w54:bool)
            n25 = Select(t=1.2, s=w54, f=0.8) -> (s? t:f=w51:dbl)
            n26 = Multiply(x=w51, y=w50) -> (x*y=w48:dbl)
            n27 = property on="Image" class="ImageControl"("X Zoom"=w48, "Y Zoom"=w48, "Image Center Position"=w49) -> ()  [unwired: 2 in, 2 out]
            n28 = call <vilib>:"Add State(s) to Queue__JKI_lib_State_Machine.vi"("State(s) in (\"\")"=w59) -> ("States Out"=w58:string)  [unwired: 14 in]
          }
          event "Well Radius": Mouse Up {
            n29 = event-data() -> ()  [unwired: 1 in, 8 out]
            n30 = call <vilib>:"Add State(s) to Queue__JKI_lib_State_Machine.vi"("State(s) in Front (\"\")"="Image: Draw\nUI: Tutorial" ("State(s) in Front (\"\")"), "State(s) in (\"\")"=w64) -> ("States Out"=w63:string)  [unwired: 13 in]
          }
          event "Fixpoint Radius": Value Change {
            n31 = event-data() -> ()  [unwired: 1 in, 6 out]
            n32 = call <vilib>:"Add State(s) to Queue__JKI_lib_State_Machine.vi"("State(s) in Front (\"\")"="Image: Draw\nUI: Tutorial" ("State(s) in Front (\"\")"), "State(s) in (\"\")"=w69) -> ("States Out"=w68:string)  [unwired: 13 in]
          }
          event "Show All Points": Value Change {
            n33 = event-data() -> ()  [unwired: 1 in, 6 out]
            n34 = call <vilib>:"Add State(s) to Queue__JKI_lib_State_Machine.vi"("State(s) in Front (\"\")"="Image: Draw" ("State(s) in Front (\"\")"), "State(s) in (\"\")"=w74) -> ("States Out"=w73:string)  [unwired: 13 in]
          }
          event "Image": Mouse Up {
            w77 = u32 1 items=["Zoom Tool"=8, "Selection Tool"=0, "Pan Tool"=9, "Point Tool"=1, "Line Tool"=2, "Rectangle Tool"=3, "Rotated Rectangle Tool"=12, "Polyline Tool"=10, "Polygon Tool"=5, "Freehand Tool"=11, "Closed Freehand Tool"=6, "Ellipse Tool"=4, "Annulus Tool"=7] ("Current ROI Tool")
            # "Timeout Frame\n(this will only execute if the Event Structure timeout is >= 0)"
            n35 = event-data() -> ()  [unwired: 1 in, 8 out]
            n36 = property on="Image" class="ImageControl"() -> ("Current ROI Tool"=w78:u32)  [unwired: 2 in, 2 out]
            n37 = Equal?(x=w78, y=w77) -> (x = y?=w76:bool)
            n38 = case shown="True" w76 {
              tunnel: w82 -> [w86 w91]
              tunnel: w81 -> [w85 w90]
              tunnel: [w85 w89] -> w80
              tunnel: [w86 w88] -> w79
              tunnel: [_ w87] -> w75
              frame False {
              }
              frame True {
                n39 = Unbundle By Name(w90) -> ("State"=w94:i32)
                n40 = property on="Image" class="ImageControl"(error in=w91) -> (error out=w92:errorcluster, "ROI"=w93:T6)  [unwired: 1 in, 1 out]
                n41 = case shown="-1, Default" w94 {
                  tunnel: w93 -> [_ w102 w109 w117 w124]
                  tunnel: w92 -> [w95 w101 w108 w116 w123]
                  tunnel: w90 -> [w96 w98 w105 w115 w122]
                  tunnel: [w96 w99 w106 w114 w121] -> w89
                  tunnel: [w95 w100 w107 w112 w119] -> w88
                  tunnel: [_ "Image: Draw\nUI: Tutorial" "Image: Draw\nUI: Tutorial" "Image: Draw\nUI: Tutorial" "Image: Draw\nUI: Tutorial"] -> w87
                  frame -1, Default {
                  }
                  frame 2 {
                    n42 = call "IMAQ Convert ROI to Point"("error in (no error)"=w101, "ROI Descriptor"=w102) -> ("error out"=w100:errorcluster, "Point"=w103:T3)  [unwired: 7 in]
                    n43 = Bundle By Name(cluster=w98, "Points.Fixpoint"=w103) -> (w99:T1)
                  }
                  frame 3 {
                    n44 = call "IMAQ Convert ROI to Point"("error in (no error)"=w108, "ROI Descriptor"=w109) -> ("error out"=w107:errorcluster, "Point"=w110:T3)  [unwired: 7 in]
                    n45 = Bundle By Name(cluster=w105, "Points.Top Left"=w110) -> (w106:T1)
                  }
                  frame 4 {
                    n46 = call "IMAQ Convert ROI to Point"("error in (no error)"=w116, "ROI Descriptor"=w117) -> ("error out"=w112:errorcluster, "Point"=w113:T3)  [unwired: 7 in]
                    n47 = Bundle By Name(cluster=w115, "Points.Top Right"=w113) -> (w114:T1)
                  }
                  frame 5 {
                    n48 = call "IMAQ Convert ROI to Point"("error in (no error)"=w123, "ROI Descriptor"=w124) -> ("error out"=w119:errorcluster, "Point"=w120:T3)  [unwired: 7 in]
                    n49 = Bundle By Name(cluster=w122, "Points.Bottom Left"=w120) -> (w121:T1)
                  }
                }
              }
            }
            n50 = call <vilib>:"Add State(s) to Queue__JKI_lib_State_Machine.vi"("State(s) in Front (\"\")"=w75, "State(s) in (\"\")"=w84) -> ("States Out"=w83:string)  [unwired: 13 in]
          }
          event "Next": Value Change {
            # "Timeout Frame\n(this will only execute if the Event Structure timeout is >= 0)"
            n51 = event-data() -> ()  [unwired: 1 in, 6 out]
            n52 = Unbundle By Name(w133) -> ("State"=w132:i32)
            n53 = Increment(x=w132) -> (x+1=w128:i32)
            n54 = In Range and Coerce(upper limit=6, x=w128, lower limit=0) -> (coerced(x)=w125:i32)  [unwired: 1 out]
            n55 = local write "State"(w125) -> ()
            n56 = Bundle By Name(cluster=w133, "State"=w125) -> (w131:T1)
            n57 = call <vilib>:"Add State(s) to Queue__JKI_lib_State_Machine.vi"("State(s) in Front (\"\")"="UI: Tutorial\nImage: Set ROI" ("f"), "State(s) in (\"\")"=w135) -> ("States Out"=w134:string)  [unwired: 13 in]
          }
          event "Previous": Value Change {
            # "Timeout Frame\n(this will only execute if the Event Structure timeout is >= 0)"
            n58 = event-data() -> ()  [unwired: 1 in, 6 out]
            n59 = Unbundle By Name(w144) -> ("State"=w143:i32)
            n60 = Decrement(x=w143) -> (x-1=w138:i32)
            n61 = In Range and Coerce(upper limit=6, x=w138, lower limit=0) -> (coerced(x)=w139:i32)  [unwired: 1 out]
            "State" <- w139
            n62 = Bundle By Name(cluster=w144, "State"=w139) -> (w142:T1)
            n63 = call <vilib>:"Add State(s) to Queue__JKI_lib_State_Machine.vi"("State(s) in Front (\"\")"="UI: Tutorial\nImage: Set ROI" ("f"), "State(s) in (\"\")"=w146) -> ("States Out"=w145:string)  [unwired: 13 in]
          }
          event Panel Close? {
            (unwired) TRUE ("Discard?")
            # "Close Panel button (pressed) Event\n(this executes Macro: Exit to terminate the VI)"
            n64 = event-data() -> ()  [unwired: 1 in, 1 out]
            n65 = event-data("Discard?"=TRUE) -> ()  [unwired: 1 in, 1 out]
            n66 = call <vilib>:"Add State(s) to Queue__JKI_lib_State_Machine.vi"("State(s) in Front (\"\")"="Macro: Exit", "State(s) in (\"\")"=w152) -> ("States Out"=w151:string)  [unwired: 13 in]
          }
          event "Done": Value Change {
            (unwired) TRUE ("Discard?")
            # "Close Panel button (pressed) Event\n(this executes Macro: Exit to terminate the VI)"
            n67 = event-data() -> ()  [unwired: 1 in, 6 out]
            n68 = call <vilib>:"Add State(s) to Queue__JKI_lib_State_Machine.vi"("State(s) in Front (\"\")"="Macro: Exit", "State(s) in (\"\")"=w157) -> ("States Out"=w156:string)  [unwired: 13 in]
          }
        }
      }
      frame "---------- Core ----------" {
        # "Do not put any code in this frame.\n(it is a separator no-op)"
        n69 = call <vilib>:"Add State(s) to Queue__JKI_lib_State_Machine.vi"("State(s) in (\"\")"=w161) -> ("States Out"=w160:string)  [unwired: 14 in]
      }
      frame Default {
        w171 = 42 items=["No error", "Argument error", "Memory is full", "Out of zone", "End of file", "File already open", "Generic file I/O error", "File not found", "File permission error", "Disk is full", "Duplicate path", "Too many files open", "System feature not enabled", "Resource file not found", "Cannot add resource", "Resource not found", "Image not found", "Image memory error", "Pen does not exist", "Config type invalid", "Config token not found", "Config parse error", "Config memory error", "Bad external code format", "Bad external code offset", "External code not present", "Null window", "Destroy window error", "Null menu", "Print aborted", "Bad print record", "Print driver error", "Windows error during printing", "Memory error during printing", "Print dialog error", "Generic print error", "Invalid device refnum", "Device not found", "Device parameter error", "Device unit error", "Cannot open device", "Device call aborted", "Generic error", "Cancelled by user", "Object ID too low", "Object ID too high", "Object not in heap", "Unknown heap", "Unknown object (invalid DefProc)", "Unknown object (DefProc not in table)", "Message out of range", "Invalid (null) method", "Unknown message", "Manager call not supported", "Bad address", "Network operation in progress", "Network operation timed out", "Connection is busy", "Network attribute not supported", "Network error", "Address in use", "System out of memory", "Connection aborted", "Connection refused", "Not connected", "Already connected", "Connection closed", "Initialization error (interapplication manager)", "Bad occurrence", "Wait on unbound occurrence handler", "Occurrence queue overflow", "Datalog type conflict", "Unused", "Unrecognized type (interapplication manager)", "Memory corrupt", "Failed to make temporary DLL", "Old CIN version", "Drag socket not found", "Failed to load drop-object", "Failed to register OLE object", "Failed to release OLE object", "Format specifier type mismatch", "Unknown format specifier", "Too few format specifiers", "Too many format specifiers", "Scan failed", "Newer CIN version", "Error converting to variant", "Runtime menu error", "Password tampered", "Variant attribute not found", "Incompatible variant data type", "Event data is not available", "Event Store is not present", "Occurrence is not found", "Event Queue is not created", "Event info is not available", "Refnum passed is NULL", "Error retrieving Class GUID", "Error retrieving CoClass GUID", "Error retrieving TypeLib GUID.", "Bad built application magic bytes.", "Specific driver is different from the specific driver associated with the Logical Name.", "There is no session opened to the class driver.", "Max Error", "MAX - Error with config objects", "MAX - Error loading configuration", "MAX - Group not supported"]
        # "Current State"
        # "Do not delete, rename, or modify this frame.\n(this is used to capture unhandled states and typos)"
        # "Handle mistyped state name (developer tool)"
        n70 = Format Into String(format string="Software Exception: Unhandled State \"%s\"." ("message"), error in=w167, w162) -> (resulting string=w170:string, error out=w169:errorcluster)  [unwired: 1 in]
        n71 = call <vilib>:"Error Cluster From Error Code.vi"("show call chain? (False)"=TRUE, "error in (no error)"=w169, "error message (\"\")"=w170, "error code (0)"=w171) -> ("error out"=w168:errorcluster)  [unwired: 5 in]
        n72 = call <vilib>:"Add State(s) to Queue__JKI_lib_State_Machine.vi"("State(s) in (\"\")"=w166) -> ("States Out"=w165:string)  [unwired: 14 in]
      }
      frame "Initialize Core Data" {
        # "Do not delete, rename, or modify this frame.\n(this is used to determine panel behavior on exit)"
        # "originally closed?"
        # "exe?"
        # "If panel starts closed or is an EXE, then close it when we exit"
        n73 = property class="App"() -> ("App.Kind"=w181:T5)  [unwired: 2 in, 2 out]
        n74 = control-ref of="Current VI Reference"() -> (w176:refnum<vi>)
        n75 = property class="VI"() -> ("FP.State"=w175:T4)  [unwired: 2 in, 2 out]
        n76 = Equal?(x=w175, y=T4."Closed" ("Front Panel Window:State")) -> (x = y?=w173:bool)
        n77 = Equal?(x=w181, y=T5."Run Time System" ("Application:Kind")) -> (x = y?=w179:bool)
        n78 = Or(x=w173, y=w179) -> (x .or. y?=w177:bool)
        n79 = Bundle By Name(cluster=w178, "Core.Current VI Reference"=w176, "Core.Close Panel on Exit?"=w177) -> (w183:T1)
        n80 = call <vilib>:"Add State(s) to Queue__JKI_lib_State_Machine.vi"("State(s) in (\"\")"=w185) -> ("States Out"=w184:string)  [unwired: 14 in]
      }
      frame "Error Handler" {
        # "Unhandled Error -- Display it"
        # "Handle any errors here.\nYou can also output any states to clean-up after errors occur"
        # "Clear error"
        n81 = call <vilib>:"General Error Handler.vi"("error in (no error)"=w187) -> ()  [unwired: 10 in, 5 out]
        n82 = call <vilib>:"Add State(s) to Queue__JKI_lib_State_Machine.vi"("State(s) in Front (\"\")"="/* Post Error States", "State(s) in (\"\")"=w191) -> ("States Out"=w190:string)  [unwired: 13 in]
      }
      frame "Exit" {
        # "Do not put any code in this frame.\n(No errors that occur here will be handled.)"
        n83 = call <vilib>:"Add State(s) to Queue__JKI_lib_State_Machine.vi"("State(s) in (\"\")"=w196) -> ("States Out"=w195:string)  [unwired: 14 in]
      }
      frame "---------- Data ----------" {
        # "Do not put any code in this frame.\n(It is a separator no-op. You can make a copy of this frame to create a new Data frame)"
        n84 = call <vilib>:"Add State(s) to Queue__JKI_lib_State_Machine.vi"("State(s) in (\"\")"=w200) -> ("States Out"=w199:string)  [unwired: 14 in]
      }
      frame "Data: Load Image" {
        # "Do not put any code in this frame.\n(It is a separator no-op. You can make a copy of this frame to create a new Data frame)"
        n85 = Empty String/Path?(string/path="Path") -> (empty?=w203:bool)
        n86 = case shown="False" w203 {
          tunnel: w205 -> [w210 w222]
          tunnel: [w219 w222] -> w201
          tunnel: "Path" -> [w218 _]
          tunnel: [w212 _] -> w202
          frame False {
            w214 = T12 7 items=["Grayscale (U8)", "Grayscale (I16)", "Grayscale (SGL)", "Complex (CSG)", "RGB (U32)", "HSL (U32)", "RGB (U64)", "Grayscale (U16)"] ("Image Type")
            n87 = call "IMAQ Create"("Image Name"="img_in", "Image Type"=w214, "error in (no error)"=w210) -> ("New Image"=w216:T2, "error out"=w217:errorcluster)  [unwired: 2 in]
            n88 = call "IMAQ ReadFile 2"("File Path"=w218, "error in (no error)"=w217, "Image"=w216) -> ("error out"=w215:errorcluster, "Image Out"=w213:T2)  [unwired: 4 in, 3 out]
            n89 = call "IMAQ Clear Overlay"("error in (no error)"=w215, "Image"=w213) -> ("error out"=w221:errorcluster, "Image Out"=w212:T2)  [unwired: 8 in]
            "Image" <- w212
            n90 = property on="Image" class="ImageControl"(error in=w221, "ROI"=T6 {"Global Rectangle"=[], "Contours"=[]}) -> (error out=w219:errorcluster)  [unwired: 1 in, 1 out]
          }
          frame True {
          }
        }
        n91 = Bundle By Name(cluster=w207, "Image Out"=w202) -> (w206:T1)
        n92 = call <vilib>:"Add State(s) to Queue__JKI_lib_State_Machine.vi"("State(s) in (\"\")"=w209) -> ("States Out"=w208:string)  [unwired: 14 in]
      }
      frame "Data: Set Image" {
        # "Do not put any code in this frame.\n(It is a separator no-op. You can make a copy of this frame to create a new Data frame)"
        n93 = Unbundle By Name(w227) -> ("img_array"=w226:T2[])
        n94 = Index Array(array=w226, index="Image") -> (element=w223:T2)
        n95 = Bundle By Name(cluster=w227, "Image Out"=w223) -> (w228:T1)
        n96 = call <vilib>:"Add State(s) to Queue__JKI_lib_State_Machine.vi"("State(s) in (\"\")"=w230) -> ("States Out"=w229:string)  [unwired: 14 in]
      }
      frame "Data: Show Img" {
        # "Do not put any code in this frame.\n(It is a separator no-op. You can make a copy of this frame to create a new Data frame)"
        n97 = Unbundle By Name(w231) -> ("Image Out"=w232:T2)
        n98 = local write "Image"(w232) -> ()
        n99 = call <vilib>:"Add State(s) to Queue__JKI_lib_State_Machine.vi"("State(s) in (\"\")"=w235) -> ("States Out"=w234:string)  [unwired: 14 in]
      }
      frame "Data: Initialize" {
        w242 = dbl[][] []  # Temps_Array
        w243 = dbl[] []  # Temps
        w244 = T2[] []  # img_array
        w238 = 0  # State
        w246 = T13 {"Current VI Reference"=refnum, "Close Panel on Exit?"=FALSE}  # Core
        # "Initialize the shift-register data, here.\n(data names are defined by what you wire into the bundle function)"
        n100 = call "TCam_Calibration_LoadSettings.vi"("error in (no error)"=w241) -> ("error out"=w240:errorcluster, "Fixpoint Area"=w236:dbl, "Scan Area"=w237:dbl, "Points"=w239:T14)  [unwired: 7 in]
        n101 = local write "Fixpoint Radius"(w236) -> ()
        n102 = local write "Well Radius"(w237) -> ()
        n103 = local write "State"(w238) -> ()
        n104 = Bundle("Core"=w246, "Image Out"=T2 refnum, "State"=w238, "Points"=w239, "img_array"=w244, "Temps"=w243, "Temps_Array"=w242) -> (w247:T15)  [unwired: 1 in]
        n105 = call <vilib>:"Add State(s) to Queue__JKI_lib_State_Machine.vi"("State(s) in (\"\")"=w249) -> ("States Out"=w248:string)  [unwired: 14 in]
      }
      frame "Data: Cleanup" {
        # "Cleanup any data and references, here.\n(this is called automatically, by the Macro: Exit)"
        n106 = Unbundle By Name(w279) -> ("Points.Top Left"=w261:T3, "Points.Top Right"=w260:T3, "Points.Bottom Left"=w259:T3, "Points.Bottom Right"=w258:T3, "Points.Fixpoint"=w254:T3, "Core.Current VI Reference"=w280:refnum<vi>)
        n107 = local read "Fixpoint Radius"() -> (w252:i32)
        n108 = local read "Well Radius"() -> (w257:u32)
        n109 = Unbundle By Name(T7 {"Core"={"Current VI Reference"=refnum, "Close Panel on Exit?"=FALSE, "Exit"=FALSE, "Initialized?"=FALSE}, "Connections"={"cDAQ Therm"={"Task"="", "Connected"=FALSE, "Active"=FALSE}, "cDAQ Voltage"={"Task"="", "Connected"=FALSE, "Active"=FALSE}, "cDAQ ID"="", "Camera"={"Session"="", "Connected"=FALSE, "Active"=FALSE, "Placeholder"=refnum}, "PSU"={"Port"="", "Connected"=FALSE, "Active"=FALSE}}, "Data Acquisition"={"Setup"={"Label"="", "Operator"="", "Notes"="", "TempGrad"=1.0, "TargetTemp"=1.0, "Sample Volume"=1.0}, "Camera"={"Image"=refnum, "Save Image"=refnum, "Image Frequency"=20, "Rectangle"={"Left"=0, "Top"=0, "Right"=0, "Bottom"=0, "Rotation"=0.0}, "Calibration"={"Top Left"={"X"=0.0, "Y"=0.0}, "Top Right"={"X"=0.0, "Y"=0.0}, "Bottom Left"={"X"=0.0, "Y"=0.0}, "Bottom Right"={"X"=0.0, "Y"=0.0}, "Fixpoint"={"X"=0.0, "Y"=0.0}, "Scan Area"=5.0, "Fixpoint Area"=0.0, "Well Pixels"=[], "Valid"=FALSE}, "FocusPos"=0, "Display Mapping"=10}, "Thermistor"={"Sample Size"=1, "Calibration"={"B0.100"=[], "R25"=[], "c"=[], "State"=[], "V_S"=5.0, "R_S"=100.0}, "Timing Mode"=14713}, "Partition"={"Data"=[], "Cell Label"="", "Cell Color"=0, "Height"=10, "Width"=16, "Grid"=[]}, "Queue"={"Size"=1, "Queue"=refnum}, "Sample Rate"=20, "Active"=FALSE, "Ready"=FALSE, "Graph Mode"=0}, "Control"={"Sample Rate"=1, "PID gains"={"proportional gain (Kc)"=1.0, "integral time (Ti, min)"=0.01, "derivative time (Td, min)"=0.0}}} ("Default values")) -> ("Data Acquisition.Camera.Calibration"=w250:T16)
        n110 = Bundle(cluster=w250, "Top Left"=w261, "Top Right"=w260, "Bottom Left"=w259, "Bottom Right"=w258, "Fixpoint"=w254, "Scan Area"=w257, "Fixpoint Area"=w252, "Well Pixels"=cluster{"X":i32, "Y":i32}[][] [], "Valid"=FALSE) -> (w262:T16)
        n111 = call <vilib>:"Application Directory.vi"() -> ("Application Directory"=w274:path)
        n112 = Path To String(path=w274) -> (string=w275:string)
        n113 = Concatenate Strings(w275, "\\TCam.ini" ("string")) -> (w272:string)
        n114 = String To Path(string=w272) -> (path=w271:path)
        n115 = call <vilib>:"Check if File or Folder Exists.vi"("error in (no error)"=w264, "path"=w271) -> ("error out"=w268:errorcluster, "file or folder exists?"=w270:bool, "dup path"=w269:path)  [unwired: 7 in]
        n116 = case shown="True" w270 {
          tunnel: w269 -> [w283 w287]
          tunnel: w268 -> [w285 w288]
          tunnel: [w284 w288] -> w267
          tunnel: [w283 w287] -> w266
          frame False {
            n117 = Open/Create/Replace File(file path (use dialog)=w283, error in=w285, operation (0:open)=T10."create") -> (error out=w284:errorcluster)  [unwired: 3 in, 2 out]
          }
          frame True {
          }
        }
        n118 = Flatten To XML(6:w262) -> (2:w265:string)
        n119 = call-poly <vilib>:"Write to XML File.vi"("error in (no error)"=w267, "XML Input"=w265, "XML File Path"=w266) -> ("error out"=w263:errorcluster)  [unwired: 6 in, 2 out]
        n120 = local read "Image"() -> (w253:T2)
        n121 = Close Reference(reference=w280, error in (no error)=w263) -> (error out=w277:errorcluster)
        n122 = call "IMAQ Dispose"("All Images? (No)"=TRUE, "Image"=w253, "error in (no error)"=w277) -> ("error out"=w276:errorcluster)  [unwired: 3 in]
        n123 = call <vilib>:"Add State(s) to Queue__JKI_lib_State_Machine.vi"("State(s) in (\"\")"=w282) -> ("States Out"=w281:string)  [unwired: 14 in]
      }
      frame "---------- UI ----------" {
        # "Do not put any code in this frame.\n(It is a separator no-op. You can make a copy of this frame to create a new UI frame)"
        n124 = call <vilib>:"Add State(s) to Queue__JKI_lib_State_Machine.vi"("State(s) in (\"\")"=w292) -> ("States Out"=w291:string)  [unwired: 14 in]
      }
      frame "UI: Initialize" {
        w293 = u32 0 items=["Grayscale", "Binary", "Gradient", "Rainbow", "Temperature", "User Defined", "Binary 16 Bit", "Gradient 16 Bit", "Rainbow 16 Bit", "Temperature 16 Bit", "User Defined 16 Bit"] ("Palette:Palette Type")
        w298 = T12 4 items=["Grayscale (U8)", "Grayscale (I16)", "Grayscale (SGL)", "Complex (CSG)", "RGB (U32)", "HSL (U32)", "RGB (U64)", "Grayscale (U16)"] ("Image Type")
        w306 = u32 1 items=["Zoom Tool"=8, "Selection Tool"=0, "Pan Tool"=9, "Point Tool"=1, "Line Tool"=2, "Rectangle Tool"=3, "Rotated Rectangle Tool"=12, "Polyline Tool"=10, "Polygon Tool"=5, "Freehand Tool"=11, "Closed Freehand Tool"=6, "Ellipse Tool"=4, "Annulus Tool"=7] ("Current ROI Tool")
        w307 = u32 15 items=["Default"=10, "Most Significant Bits"=11, "Full Dynamic"=12, "Downshift"=13, "Given Range"=14, "90% Dynamic"=15, "Given Percent Range"=16] ("16-bit Display Mapping:Conversion Method")
        # "Initialize the User Interface, here.\n(this is called automatically, by the Macro: Init)"
        n125 = call <vilib>:"Application Directory.vi"() -> ("Application Directory"=w302:path)
        n126 = Path To String(path=w302) -> (string=w304:string)
        n127 = call "IMAQ Create"("Image Name"="placeholder_img", "Image Type"=w298) -> ("New Image"=w301:T2)  [unwired: 3 in, 1 out]
        n128 = Concatenate Strings(w304, "\\resources\\camera_placeholder.png") -> (w303:string)
        n129 = String To Path(string=w303) -> (path=w305:path)
        n130 = call "IMAQ ReadFile 2"("Use File Path Image Type"=FALSE, "File Path"=w305, "Image"=w301) -> ("Image Out"=w296:T2)  [unwired: 4 in, 4 out]
        n131 = property on="Image" class="ImageControl"("16-bit Display Conversion Method"=w307) -> ()  [unwired: 2 in, 2 out]
        n132 = property on="Image" class="ImageControl"("Current ROI Tool"=w306, "Palette Type"=w293) -> ()  [unwired: 2 in, 2 out]
        n133 = local write "Display Mapping"(w307) -> ()
        n134 = local write "Image"(w296) -> ()
        n135 = local write "Path"(path "" ("Path")) -> ()
        n136 = property on="Image" class="ImageControl"("Zoom to Fit Mode"=TRUE) -> ()  [unwired: 2 in, 2 out]
        n137 = call <vilib>:"Add State(s) to Queue__JKI_lib_State_Machine.vi"("State(s) in Front (\"\")"="UI: Tutorial\n// UI: Progress >> Hide" ("State(s) in Front (\"\")"), "State(s) in (\"\")"=w312) -> ("States Out"=w311:string)  [unwired: 13 in]
      }
      frame "UI: Tutorial" {
        # "Initialize the User Interface, here.\n(this is called automatically, by the Macro: Init)"
        n138 = local read "State"() -> (w327:i32)
        n139 = case shown="0, Default" w327 {
          tunnel: ["Load Calibration Image." "Select a Display Mapping that shows a clear image.\n\nSelect correct PCR size." w346 w363 w369 w375 "Select Well Radius so the center of each well is covered.\n\nGo to previous steps to adjust positions. Press done once satisfied."] -> w326
          tunnel: [_ _ _ _ _ _ w378] -> w325
          tunnel: [_ _ _ _ _ _ w378] -> w324
          tunnel: [_ w339 _ _ _ _ _] -> w323
          tunnel: [_ w339 _ _ _ _ _] -> w322
          tunnel: [w331 w339 w347 w359 w365 w371 _] -> w321
          tunnel: [_ w339 w353 TRUE TRUE TRUE w378] -> w320
          tunnel: [TRUE _ _ _ _ _ _] -> w319
          tunnel: [_ _ w344 _ _ _ _] -> w318
          tunnel: w317 -> [_ _ w356 w360 w366 w372 _]
          tunnel: ["Step: 1/7" "Step: 2/7" "Step: 3/7" "Step: 4/7" "Step: 5/7" "Step: 6/7" "Step: 7/7"] -> w316
          tunnel: [_ _ _ _ _ _ w376] -> w315
          tunnel: [_ TRUE w353 _ _ _ _] -> w314
          tunnel: [_ 0 ("t") w350 _ _ _ _] -> w313
          frame 0, Default {
            n140 = local read "Path"() -> (w333:path)
            n141 = Empty String/Path?(string/path=w333) -> (empty?=w332:bool)
            n142 = Not(x=w332) -> (.not. x?=w331:bool)
          }
          frame 1 {
            w339 = TRUE
          }
          frame 2 {
            w353 = TRUE
            w357 = "Select Fix Point Cavity (Left Click) as shown (zoom with Mouse Wheel).\n\nYou can move the point by Left Click and dragging.\n\n"  # Select Fix Point Cavity (Left Click) as shown (zoom with Mouse Wheel).  You can move the point by Left Click and dragging.
            n143 = Unbundle By Name(w356) -> ("Points.Fixpoint.X"=w355:sgl)
            n144 = local read "Fixpoint Radius"() -> (w349:i32)
            n145 = Not Equal To 0?(x=w355) -> (x != 0?=w344:bool)
            n146 = Not Equal To 0?(x=w349) -> (x != 0?=w348:bool)
            n147 = And(x=w348, y=w344) -> (x .and. y?=w347:bool)
            n148 = Select(t="Set Fixpoint Radius so the cavity is appropriately filled as shown. ", s=w344, f="") -> (s? t:f=w345:string)
            n149 = Select(t=2, s=w344, f=1) -> (s? t:f=w350:i32)
            n150 = Concatenate Strings(w357, w345) -> (w346:string)
          }
          frame 3 {
            w363 = "Select Top Left corner of PCR plate as shown."  # Select Top Left corner of PCR plate as shown.
            n151 = Unbundle By Name(w360) -> ("Points.Top Left.X"=w361:sgl)
            n152 = Not Equal To 0?(x=w361) -> (x != 0?=w359:bool)
          }
          frame 4 {
            w369 = "Select Top Right corner of PCR plate as shown."  # Select Top Right corner of PCR plate as shown.
            n153 = Unbundle By Name(w366) -> ("Points.Top Right.X"=w367:sgl)
            n154 = Not Equal To 0?(x=w367) -> (x != 0?=w365:bool)
          }
          frame 5 {
            w375 = "Select Bottom Left corner of PCR plate as shown."  # Select Bottom Left corner of PCR plate as shown.
            n155 = Unbundle By Name(w372) -> ("Points.Bottom Left.X"=w373:sgl)
            n156 = Not Equal To 0?(x=w373) -> (x != 0?=w371:bool)
          }
          frame 6 {
            w378 = TRUE
            n157 = local read "Well Radius"() -> (w377:u32)
            n158 = Not Equal To 0?(x=w377) -> (x != 0?=w376:bool)
          }
        }
        "Tutorial" <- w326
        "Step" <- w316
        "Pict Ring" <- w313
        n159 = property on="Fixpoint Radius" class="DigNum (strict)"("Visible"=w318) -> ()  [unwired: 2 in, 2 out]
        n160 = property on="Path" class="Path"("Visible"=w319) -> ()  [unwired: 2 in, 2 out]
        n161 = property on="Well Radius" class="DigNum (strict)"("Visible"=w325) -> ()  [unwired: 2 in, 2 out]
        n162 = property on="Show All Points" class="Bool (strict)"("Visible"=w324) -> ()  [unwired: 2 in, 2 out]
        n163 = property on="Display Mapping" class="Ring (strict)"("Visible"=w323) -> ()  [unwired: 2 in, 2 out]
        n164 = property on="PCR Size" class="Ring (strict)"("Visible"=w322) -> ()  [unwired: 2 in, 2 out]
        n165 = property on="Next" class="Bool"("Visible"=w321) -> ()  [unwired: 2 in, 2 out]
        n166 = property on="Previous" class="Bool"("Visible"=w320) -> ()  [unwired: 2 in, 2 out]
        n167 = property on="Done" class="Bool"("Visible"=w315) -> ()  [unwired: 2 in, 2 out]
        n168 = property on="Pict Ring" class="Ring (strict)"("Visible"=w314) -> ()  [unwired: 2 in, 2 out]
        n169 = call <vilib>:"Add State(s) to Queue__JKI_lib_State_Machine.vi"("State(s) in (\"\")"=w330) -> ("States Out"=w329:string)  [unwired: 14 in]
      }
      frame "UI: Cursor Set" {
        # "Argument"
        # "Set and Unset Cursor Busy.\n(Usage: \"UI: Cursor Set >> Busy|Idle\")"
        n170 = case shown="\"Busy\"" w381 {
          tunnel: w383 -> [w388 w390]
          tunnel: [w387 w389] -> w382
          frame "Idle", Default {
            n171 = call <vilib>:"Unset Busy.vi"("error in (no error)"=w388) -> ("error out"=w387:errorcluster)  [unwired: 10 in]
          }
          frame "Busy" {
            n172 = call <vilib>:"Set Busy.vi"("error in (no error)"=w390) -> ("error out"=w389:errorcluster)  [unwired: 9 in, 1 out]
          }
        }
        n173 = call <vilib>:"Add State(s) to Queue__JKI_lib_State_Machine.vi"("State(s) in (\"\")"=w386) -> ("States Out"=w385:string)  [unwired: 14 in]
      }
      frame "UI: Front Panel State" {
        # "Argument"
        # "Set Front Panel Open or Closed\n(Usage: \"UI: Front Panel State >> Open|Close\")"
        n174 = Unbundle By Name(w393) -> ("Core.Current VI Reference"=w392:refnum<vi>)
        n175 = case shown="\"Minimize\", \"Minimized\"" w391 {
          tunnel: w395 -> [w403 w418 w429 w442 w455]
          tunnel: [w405 w419 w431 w444 w457] -> w394
          tunnel: w392 -> [w404 w416 w430 w443 w456]
          frame "Open", "Standard", Default {
            w398 = T4."Standard" ("State")
            n176 = property class="VI"(reference=w404, error in=w403) -> (reference out=w401:refnum<vi>, error out=w402:errorcluster, "FP.State"=w400:T4)
            n177 = Not Equal?(x=w400, y=w398) -> (x != y?=w399:bool)
            n178 = case shown="True" w399 {
              tunnel: [w409 w411] -> w405
              tunnel: w402 -> [w408 w411]
              tunnel: w401 -> [w407 _]
              tunnel: w398 -> [w406 _]
              frame True {
                n179 = invoke class="VI" method="FP.Open"(reference=w407, error in=w408, "Activate"=TRUE, "State"=w406) -> (error out=w409:errorcluster)  [unwired: 1 in, 4 out]
              }
              frame False {
              }
            }
          }
          frame "Close", "Closed" {
            n180 = property class="VI"(reference=w416, error in=w418) -> (reference out=w415:refnum<vi>, error out=w417:errorcluster, "FP.State"=w413:T4)
            n181 = Not Equal?(x=w413, y=T4."Closed" ("Front Panel Window:State")) -> (x != y?=w412:bool)
            n182 = case shown="True" w412 {
              tunnel: [w420 w423] -> w419
              tunnel: w417 -> [w420 w422]
              tunnel: w415 -> [_ w421]
              frame False {
              }
              frame True {
                n183 = invoke class="VI" method="FP.Close"(reference=w421, error in=w422) -> (error out=w423:errorcluster)  [unwired: 1 in, 2 out]
              }
            }
          }
          frame "Hidden", "Hide" {
            w424 = T4."Hidden" ("State")
            n184 = property class="VI"(reference=w430, error in=w429) -> (reference out=w427:refnum<vi>, error out=w428:errorcluster, "FP.State"=w426:T4)
            n185 = Not Equal?(x=w426, y=w424) -> (x != y?=w425:bool)
            n186 = case shown="True" w425 {
              tunnel: [w435 w436] -> w431
              tunnel: w428 -> [w434 w436]
              tunnel: w427 -> [w433 _]
              tunnel: w424 -> [w432 _]
              frame True {
                n187 = invoke class="VI" method="FP.Open"(reference=w433, error in=w434, "State"=w432) -> (error out=w435:errorcluster)  [unwired: 2 in, 4 out]
              }
              frame False {
              }
            }
          }
          frame "Minimize", "Minimized" {
            w437 = T4."Minimized" ("State")
            n188 = property class="VI"(reference=w443, error in=w442) -> (reference out=w440:refnum<vi>, error out=w441:errorcluster, "FP.State"=w439:T4)
            n189 = Not Equal?(x=w439, y=w437) -> (x != y?=w438:bool)
            n190 = case shown="True" w438 {
              tunnel: [w448 w449] -> w444
              tunnel: w441 -> [w447 w449]
              tunnel: w440 -> [w446 _]
              tunnel: w437 -> [w445 _]
              frame True {
                n191 = invoke class="VI" method="FP.Open"(reference=w446, error in=w447, "State"=w445) -> (error out=w448:errorcluster)  [unwired: 2 in, 4 out]
              }
              frame False {
              }
            }
          }
          frame "Maximize", "Maximized" {
            w450 = T4."Maximized" ("State")
            n192 = property class="VI"(reference=w456, error in=w455) -> (reference out=w453:refnum<vi>, error out=w454:errorcluster, "FP.State"=w452:T4)
            n193 = Not Equal?(x=w452, y=w450) -> (x != y?=w451:bool)
            n194 = case shown="True" w451 {
              tunnel: [w461 w462] -> w457
              tunnel: w454 -> [w460 w462]
              tunnel: w453 -> [w459 _]
              tunnel: w450 -> [w458 _]
              frame True {
                n195 = invoke class="VI" method="FP.Open"(reference=w459, error in=w460, "State"=w458) -> (error out=w461:errorcluster)  [unwired: 2 in, 4 out]
              }
              frame False {
              }
            }
          }
        }
        n196 = call <vilib>:"Add State(s) to Queue__JKI_lib_State_Machine.vi"("State(s) in (\"\")"=w397) -> ("States Out"=w396:string)  [unwired: 14 in]
      }
      frame "---------- Macro ----------" {
        # "Do not put any code in this frame.\n(It is a separator no-op. You can make a copy of this frame to create a new Macro frame)"
        n197 = call <vilib>:"Add State(s) to Queue__JKI_lib_State_Machine.vi"("State(s) in (\"\")"=w466) -> ("States Out"=w465:string)  [unwired: 14 in]
      }
      frame "Macro: Initialize" {
        w467 = "// UI: Cursor Set >> Busy\nData: Initialize\nInitialize Core Data\nUI: Initialize\nUI: Front Panel State >> Open\nUI: Tutorial\n// Image: Draw\n// UI: Cursor Set >> Idle"  # // UI: Cursor Set >> Busy Data: Initialize Initialize Core Data UI: Initialize UI: Front Panel State >> Open UI: Tutorial // Image: Draw // UI: Cursor Set >> Idle
        # "Initialization Macro\n(This is called once, when the VI starts)"
        n198 = call <vilib>:"Add State(s) to Queue__JKI_lib_State_Machine.vi"("State(s) in Front (\"\")"=w467, "State(s) in (\"\")"=w471) -> ("States Out"=w470:string)  [unwired: 13 in]
      }
      frame "Macro: Exit" {
        # "Exit Macro\n(This is called once, when the VI exits)"
        n199 = Unbundle By Name(w478) -> ("Core.Close Panel on Exit?"=w477:bool)
        n200 = Select(t="UI: Front Panel State >> Close", s=w477, f="") -> (s? t:f=w474:string)
        n201 = call <vilib>:"Add State(s) to Queue__JKI_lib_State_Machine.vi"("State(s) in (\"\")"=w474, "State(s) at Back (\"\")"="Data: Cleanup\nExit") -> ("States Out"=w472:string)  [unwired: 13 in]
        n202 = call <vilib>:"Add State(s) to Queue__JKI_lib_State_Machine.vi"("State(s) in Front (\"\")"=w472, "State(s) in (\"\")"=w481) -> ("States Out"=w480:string)  [unwired: 13 in]
      }
      frame "---------- Image ----------" {
        # "Template Separator\n(You can make a copy of, or modify, this frame)"
        n203 = call <vilib>:"Add State(s) to Queue__JKI_lib_State_Machine.vi"("State(s) in (\"\")"=w485) -> ("States Out"=w484:string)  [unwired: 14 in]
      }
      frame "Image: Draw" {
        # "Template Separator\n(You can make a copy of, or modify, this frame)"
        n204 = call <vilib>:"Add State(s) to Queue__JKI_lib_State_Machine.vi"("State(s) in Front (\"\")"="UI: Cursor Set >> Busy\nImage: Clear ROI\nImage: Set ROI\nImage: Draw Fixedpoint\nImage: Calculate BR\nImage: Calculate y space\nImage: Calculate x space\nImage: Calculate Positions\nImage: Drawlines\nImage: Draw Points\nUI: Cursor Set >> Idle" ("State(s) in Front (\"\")"), "State(s) in (\"\")"=w490) -> ("States Out"=w489:string)  [unwired: 13 in]
      }
      frame "Image: Redraw" {
        # "Template Separator\n(You can make a copy of, or modify, this frame)"
        n205 = call <vilib>:"Add State(s) to Queue__JKI_lib_State_Machine.vi"("State(s) in Front (\"\")"="UI: Cursor Set >> Busy\nImage: Clear ROI\nImage: Drawlines\nImage: Draw Points\nImage: Calculate Temps\nUI: Cursor Set >> Idle" ("State(s) in Front (\"\")"), "State(s) in (\"\")"=w495) -> ("States Out"=w494:string)  [unwired: 13 in]
      }
      frame "Image: Drawlines" {
        # "Template Separator\n(You can make a copy of, or modify, this frame)"
        n206 = Unbundle By Name(w496) -> ("Points.Top Left.X"=w512:sgl, "Points.Top Right.X"=w511:sgl, "Points.Bottom Left.X"=w510:sgl, "Points.Bottom Right.X"=w509:sgl)
        n207 = Equal To 0?(x=w509) -> (x = 0?=w499:bool)
        n208 = Equal To 0?(x=w510) -> (x = 0?=w498:bool)
        n209 = Or(x=w498, y=w499) -> (x .or. y?=w497:bool)
        n210 = Equal To 0?(x=w512) -> (x = 0?=w508:bool)
        n211 = Equal To 0?(x=w511) -> (x = 0?=w507:bool)
        n212 = Select(t="", s=w498, f="Image: Draw Line >> TL_BL\n") -> (s? t:f=w504:string)
        n213 = Select(t="", s=w497, f="Image: Draw Line >> TR_BR\nImage: Draw Line >> BL_BR\nImage: Draw Line >> Vertical\nImage: Draw Line >> Horizontal") -> (s? t:f=w501:string)
        n214 = case shown="False" w508 {
          tunnel: w507 -> [w519 _]
          tunnel: w504 -> [w518 _]
          tunnel: w501 -> [w517 _]
          tunnel: [w516 _] -> w500
          frame False {
            n215 = case shown="False" w519 {
              tunnel: w518 -> [w522 _]
              tunnel: w517 -> [w521 _]
              tunnel: [w520 _] -> w516
              frame False {
                n216 = Concatenate Strings("Image: Draw Line >> TL_TR\n", w522, w521) -> (w520:string)
              }
              frame True {
              }
            }
          }
          frame True {
          }
        }
        n217 = call <vilib>:"Add State(s) to Queue__JKI_lib_State_Machine.vi"("State(s) in Front (\"\")"=w500, "State(s) in (\"\")"=w515) -> ("States Out"=w514:string)  [unwired: 13 in]
      }
      frame "Image: Draw Fixedpoint" {
        # "Template Separator\n(You can make a copy of, or modify, this frame)"
        n218 = Unbundle By Name(w530) -> ("Image Out"=w527:T2, "Points.Fixpoint"=w529:T3)
        n219 = Build Array(w529) -> (w528:T3[])
        n220 = call "TCam_CenterArray.vi"("Size"="Fixpoint Radius", "Point Array"=w528, "Image in"=w527) -> ("Image"=w526:T2)  [unwired: 3 in, 1 out]
        n221 = local write "Image"(w526) -> ()
        n222 = call <vilib>:"Add State(s) to Queue__JKI_lib_State_Machine.vi"("State(s) in (\"\")"=w532) -> ("States Out"=w531:string)  [unwired: 14 in]
      }
      frame "Image: Clear ROI" {
        # "Your code here.\n(You can make a copy of, or modify, this frame)"
        n223 = Unbundle By Name(w536) -> ("Image Out"=w535:T2)
        n224 = call "IMAQ Clear Overlay"("error in (no error)"=w534, "Image"=w535) -> ("error out"=w533:errorcluster)  [unwired: 8 in, 1 out]
        n225 = call <vilib>:"Add State(s) to Queue__JKI_lib_State_Machine.vi"("State(s) in (\"\")"=w538) -> ("States Out"=w537:string)  [unwired: 14 in]
      }
      frame "Image: Calculate x space" {
        # "Your code here.\n(You can make a copy of, or modify, this frame)"
        n226 = Unbundle By Name(w547) -> ("Points.Top Left"=w553:T3, "Points.Top Right"=w552:T3)
        n227 = case shown="1" "PCR Size" {
          tunnel: [24 12] -> w539
          frame 0, Default {
          }
          frame 1 {
          }
        }
        n228 = Unbundle(w552) -> ("X"=w551:sgl, "Y"=w549:sgl)
        n229 = Unbundle(w553) -> ("X"=w550:sgl, "Y"=w548:sgl)
        n230 = Subtract(x=w551, y=w550) -> (x-y=w544:sgl)
        n231 = Decrement(x=w539) -> (x-1=w543:i32)
        n232 = Subtract(x=w549, y=w548) -> (x-y=w542:sgl)
        n233 = Divide(x=w544, y=w543) -> (x/y=w545:sgl)
        n234 = Divide(x=w542, y=w543) -> (x/y=w541:sgl)
        n235 = Bundle By Name(cluster=w547, "Points.x_space"=w545, "Points.y_space"=w541) -> (w546:T1)
        n236 = call <vilib>:"Add State(s) to Queue__JKI_lib_State_Machine.vi"("State(s) in (\"\")"=w556) -> ("States Out"=w555:string)  [unwired: 14 in]
      }
      frame "Image: Calculate BR" {
        # "Your code here.\n(You can make a copy of, or modify, this frame)"
        n237 = Unbundle By Name(w567) -> ("Points.Top Left"=w573:T3, "Points.Top Right"=w572:T3, "Points.Bottom Left"=w565:T3)
        n238 = Unbundle(w573) -> ("X"=w570:sgl, "Y"=w568:sgl)
        n239 = Unbundle(w572) -> ("X"=w571:sgl, "Y"=w569:sgl)
        n240 = Unbundle(w565) -> ("X"=w564:sgl, "Y"=w562:sgl)
        n241 = Subtract(x=w571, y=w570) -> (x-y=w563:sgl)
        n242 = Subtract(x=w569, y=w568) -> (x-y=w561:sgl)
        n243 = Add(x=w564, y=w563) -> (x+y=w559:sgl)
        n244 = Add(x=w561, y=w562) -> (x+y=w560:sgl)
        n245 = Bundle By Name(cluster=w567, "Points.Bottom Right.X"=w559, "Points.Bottom Right.Y"=w560) -> (w566:T1)
        n246 = call <vilib>:"Add State(s) to Queue__JKI_lib_State_Machine.vi"("State(s) in (\"\")"=w576) -> ("States Out"=w575:string)  [unwired: 14 in]
      }
      frame "Image: Calculate y space" {
        # "Your code here.\n(You can make a copy of, or modify, this frame)"
        n247 = local read "PCR Size"() -> (w578:u16)
        n248 = Unbundle By Name(w585) -> ("Points.Top Left"=w591:T3, "Points.Bottom Left"=w590:T3)
        n249 = case shown="1" w578 {
          tunnel: [16 8] -> w577
          frame 0, Default {
          }
          frame 1 {
          }
        }
        n250 = Unbundle(w590) -> ("X"=w589:sgl, "Y"=w587:sgl)
        n251 = Unbundle(w591) -> ("X"=w588:sgl, "Y"=w586:sgl)
        n252 = Subtract(x=w589, y=w588) -> (x-y=w582:sgl)
        n253 = Decrement(x=w577) -> (x-1=w581:i32)
        n254 = Subtract(x=w587, y=w586) -> (x-y=w580:sgl)
        n255 = Divide(x=w582, y=w581) -> (x/y=w583:sgl)
        n256 = Divide(x=w580, y=w581) -> (x/y=w579:sgl)
        n257 = Bundle By Name(cluster=w585, "Points.x space 2"=w583, "Points.y space 2"=w579) -> (w584:T1)
        n258 = call <vilib>:"Add State(s) to Queue__JKI_lib_State_Machine.vi"("State(s) in (\"\")"=w594) -> ("States Out"=w593:string)  [unwired: 14 in]
      }
      frame "Image: Set ROI" {
        # "Your code here.\n(You can make a copy of, or modify, this frame)"
        n259 = Unbundle By Name(w603) -> ("State"=w601:i32)
        n260 = case shown="2..5" w601 {
          tunnel: w601 -> [_ w615]
          tunnel: w603 -> [_ w613]
          tunnel: w602 -> [w608 w612]
          tunnel: [w608 w611] -> w600
          tunnel: [T11 {"Global Rectangle"=[], "Contours"=[]} ("ROI Descriptor") w610] -> w599
          tunnel: [w606 w609] -> w597
          frame 0, Default {
            w606 = u32 0 items=["Zoom Tool"=8, "Selection Tool"=0, "Pan Tool"=9, "Point Tool"=1, "Line Tool"=2, "Rectangle Tool"=3, "Rotated Rectangle Tool"=12, "Polyline Tool"=10, "Polygon Tool"=5, "Freehand Tool"=11, "Closed Freehand Tool"=6, "Ellipse Tool"=4, "Annulus Tool"=7] ("Current ROI Tool")
          }
          frame 2..5 {
            w609 = u32 1 items=["Zoom Tool"=8, "Selection Tool"=0, "Pan Tool"=9, "Point Tool"=1, "Line Tool"=2, "Rectangle Tool"=3, "Rotated Rectangle Tool"=12, "Polyline Tool"=10, "Polygon Tool"=5, "Freehand Tool"=11, "Closed Freehand Tool"=6, "Ellipse Tool"=4, "Annulus Tool"=7] ("Current ROI Tool")
            n261 = case shown="5" w615 {
              tunnel: [w617 w619 w621 w623] -> w614
              tunnel: w613 -> [w616 w618 w620 w622]
              frame 2, Default {
                n262 = Unbundle By Name(w616) -> ("Points.Fixpoint"=w617:T3)
              }
              frame 3 {
                n263 = Unbundle By Name(w618) -> ("Points.Top Left"=w619:T3)
              }
              frame 4 {
                n264 = Unbundle By Name(w620) -> ("Points.Top Right"=w621:T3)
              }
              frame 5 {
                n265 = Unbundle By Name(w622) -> ("Points.Bottom Left"=w623:T3)
              }
            }
            n266 = call "IMAQ Convert Point to ROI"("error in (no error)"=w612, "Point"=w614) -> ("error out"=w611:errorcluster, "ROI Descriptor"=w610:T11)  [unwired: 7 in]
          }
        }
        n267 = property on="Image" class="ImageControl"("Current ROI Tool"=w597) -> ()  [unwired: 2 in, 2 out]
        n268 = property on="Image" class="ImageControl"(error in=w600, "ROI"=w599) -> (error out=w598:errorcluster)  [unwired: 1 in, 1 out]
        n269 = call <vilib>:"Add State(s) to Queue__JKI_lib_State_Machine.vi"("State(s) in (\"\")"=w605) -> ("States Out"=w604:string)  [unwired: 14 in]
      }
      frame "Image: Draw Line" {
        w624 = u32 1  # Width_Minor
        w625 = u32 2  # Width
        # "Your code here.\n(You can make a copy of, or modify, this frame)"
        n270 = Unbundle By Name(w629) -> ("Image Out"=w630:T2)
        n271 = case shown="\"Vertical\"" w631 {
          tunnel: w630 -> [w635 w643 w652 w660 w667 w672 w681]
          tunnel: w629 -> [_ w644 w653 w655 w662 w676 w685]
          tunnel: [w635 w638 w651 w659 w666 w668 w677] -> w628
          tunnel: w627 -> [w634 w642 w650 w658 w665 w670 w680]
          tunnel: [w634 w637 w649 w657 w664 w669 w679] -> w626
          tunnel: w625 -> [_ w636 w645 _ _ w671 w678]
          tunnel: w624 -> [_ _ _ w654 w661 _ _]
          frame "False", Default {
          }
          frame "TL_TR" {
            n272 = Unbundle By Name(w644) -> ("Points.Top Left"=w641:T3, "Points.Top Right"=w640:T3)
            n273 = Build Array(w641, w640) -> (w639:T3[])
            n274 = call "IMAQ Overlay Multiple Lines 2"("Image"=w643, "Line End Points"=w639, "error in (no error)"=w642, "Width"=w636) -> ("Image Out"=w638:T2, "error out"=w637:errorcluster)  [unwired: 10 in]
          }
          frame "TL_BL" {
            n275 = Unbundle By Name(w653) -> ("Points.Top Left"=w648:T3, "Points.Bottom Left"=w647:T3)
            n276 = Build Array(w648, w647) -> (w646:T3[])
            n277 = call "IMAQ Overlay Multiple Lines 2"("Image"=w652, "Line End Points"=w646, "error in (no error)"=w650, "Width"=w645) -> ("Image Out"=w651:T2, "error out"=w649:errorcluster)  [unwired: 10 in]
          }
          frame "Vertical" {
            n278 = local read "PCR Size"() -> (w656:u16)
            n279 = call "TCam_VerticalLines.vi"("Width"=w654, "error in (no error)"=w658, "Cluster"=w655, "Size"=w656, "Refnum in"=w660) -> ("error out"=w657:errorcluster, "Refnum out"=w659:T2)  [unwired: 5 in]
          }
          frame "Horizontal" {
            n280 = local read "PCR Size"() -> (w663:u16)
            n281 = call "TCam_HorizontalLines.vi"("Width"=w661, "error in (no error)"=w665, "Cluster"=w662, "Size"=w663, "Refnum in"=w667) -> ("error out"=w664:errorcluster, "Refnum out"=w666:T2)  [unwired: 5 in]
          }
          frame "TR_BR" {
            n282 = Unbundle By Name(w676) -> ("Points.Top Right"=w675:T3, "Points.Bottom Right"=w674:T3)
            n283 = Build Array(w675, w674) -> (w673:T3[])
            n284 = call "IMAQ Overlay Multiple Lines 2"("Image"=w672, "Line End Points"=w673, "error in (no error)"=w670, "Width"=w671) -> ("Image Out"=w668:T2, "error out"=w669:errorcluster)  [unwired: 10 in]
          }
          frame "BL_BR" {
            n285 = Unbundle By Name(w685) -> ("Points.Bottom Left"=w684:T3, "Points.Bottom Right"=w683:T3)
            n286 = Build Array(w684, w683) -> (w682:T3[])
            n287 = call "IMAQ Overlay Multiple Lines 2"("Image"=w681, "Line End Points"=w682, "error in (no error)"=w680, "Width"=w678) -> ("Image Out"=w677:T2, "error out"=w679:errorcluster)  [unwired: 10 in]
          }
        }
        n288 = local write "Image"(w628) -> ()
        n289 = call <vilib>:"Add State(s) to Queue__JKI_lib_State_Machine.vi"("State(s) in (\"\")"=w633) -> ("States Out"=w632:string)  [unwired: 14 in]
      }
      frame "Image: Draw Points" {
        # "Your code here.\n(You can make a copy of, or modify, this frame)"
        n290 = Unbundle By Name(w687) -> ("Points.Top Left.X"=w696:sgl, "Points.Top Right.X"=w695:sgl, "Points.Bottom Left.X"=w694:sgl, "Points.Bottom Right.X"=w693:sgl)
        n291 = Equal To 0?(x=w696) -> (x = 0?=w692:bool)
        n292 = Equal To 0?(x=w695) -> (x = 0?=w691:bool)
        n293 = Equal To 0?(x=w694) -> (x = 0?=w690:bool)
        n294 = Equal To 0?(x=w693) -> (x = 0?=w689:bool)
        n295 = Unbundle By Name(w687) -> ("Image Out"=w698:T2)
        n296 = Compound Arithmetic op=OR(w692, w691, w690, w689) -> (w688:bool)
        n297 = case shown="False" w688 {
          tunnel: w698 -> [w708 _]
          tunnel: w687 -> [w703 w709]
          tunnel: [w701 w709] -> w686
          frame False {
            n298 = local read "Points"() -> (w707:T3[])
            n299 = call "TCam_CenterArray.vi"("draw all?"="Show All Points", "Size"="Well Radius", "Point Array"=w707, "Image in"=w708) -> ("Array"=w702:cluster{"X":i32, "Y":i32}[][], "Image"=w705:T2)  [unwired: 2 in]
            n300 = local write "Image"(w705) -> ()
            n301 = Bundle By Name(cluster=w703, "Points.Pixels"=w702) -> (w701:T1)
          }
          frame True {
          }
        }
        n302 = call <vilib>:"Add State(s) to Queue__JKI_lib_State_Machine.vi"("State(s) in (\"\")"=w700) -> ("States Out"=w699:string)  [unwired: 14 in]
      }
      frame "Image: Calculate Positions" {
        # "Your code here.\n(You can make a copy of, or modify, this frame)"
        n303 = Unbundle By Name(w711) -> ("Points.Top Left.X"=w719:sgl, "Points.Top Right.X"=w718:sgl, "Points.Bottom Left.X"=w717:sgl, "Points.Bottom Right.X"=w716:sgl)
        n304 = Equal To 0?(x=w719) -> (x = 0?=w715:bool)
        n305 = Equal To 0?(x=w718) -> (x = 0?=w714:bool)
        n306 = Equal To 0?(x=w717) -> (x = 0?=w713:bool)
        n307 = Equal To 0?(x=w716) -> (x = 0?=w712:bool)
        n308 = Compound Arithmetic op=OR(w715, w714, w713, w712) -> (w710:bool)
        n309 = case shown="False" w710 {
          tunnel: w711 -> [w723 _]
          frame False {
            n310 = local read "PCR Size"() -> (w724:u16)
            n311 = call "TCam_PointCalculator.vi"("Cluster"=w723, "Size"=w724) -> ("Points"=→"Points":T3[])  [unwired: 9 in]
          }
          frame True {
          }
        }
        n312 = call <vilib>:"Add State(s) to Queue__JKI_lib_State_Machine.vi"("State(s) in (\"\")"=w722) -> ("States Out"=w721:string)  [unwired: 14 in]
      }
    }
  }
  "State out" <- "Data: Load Thermal Calibration"
